vi "find.vi"() -> ()   [LabVIEW 2013]
uses:
  newCore/Variables/GlobalConAxisPI.vi
  newCore/Camera/lib/System Files/user.lib/atmcd32d.llb/Shutter_type typedef.ctl
  newCore/Camera/lib/System Files/user.lib/atmcd32d.llb/Shutter_mode typedef.ctl
  newCore/Camera/vi/GlobalSetGetConfigureCamera.vi
  newCore/Camera/vi/ccdChipPixels.vi
  <vilib>/vision/Image Controls.llb/IMAQ Rounding Mode.ctl
  newCore/Variables/patternImg.vi
  <vilib>/vision/Pattern Matching.llb/IMAQ Match Range Setting.ctl
  <vilib>/vision/Pattern Matching.llb/IMAQ Curve Parameters.ctl
panel:
  in  "Tab Control":T1(tab)
  out "Histogram":i32[][](graph)
  out "Trace":i32[][](graph)=[[2, 0, 0, 1, 1, 1, 0, 0, 0, 1, 0, 1, 0, 1, 2, 2, 0, 3, 0, 2, 2, 1, 3, 1, 0, 1, 1, 1, 0, 1, 3, 1, 0, 2, 0, 1, 0, 1, 1, 0, 1, 1, 3, 1, 0, 2, 0, 1, 1, 0, 0, 2, 0, 0, 1, 1, 1, 0, 0, 1, 0, 1, 0, 0, 0, 1, 2, 1, 1, 2, 0, 2, 4, 3, 1, 1, 0, 0, 1, 1, 2, 0, 1, 1, 0, 0, 0, 1, 1, 1, 1, 3, 0, 0, 1, 0, 0, 0, 2, 1, 1, 1, 2, 1, 0, 1, 1, 0, 0, 2, 1, 1, 0, 0, 1, 1, 1, 1, 0, 2, 2, 0, 1, 2, 1, 0, 3, 0, 2, 1, 3, 0, 1, 1, 0, 0, 3, 0, 0, 0, 0, 0, 0, 0, 0, 0, 0, 0, 0, 0, 0, 0, 0, 0, 0, 0, 0, 0, 0, 0, 0, 0, 0, 0, 0, 0, 0, 0, 0, 0, 0, 0, 0, 0, 0, 0, 0, 0, 0, 0, 0, 0, 0, 0, 0, 0, 0, 0, 0, 0, 0, 0, 0, 0, 0, 0, 0, 0, 0, 0], [1, 2, 2, 0, 0, 0, 1, 2, 1, 2, 1, 1, 1, 0, 0, 0, 3, 1, 0, 1, 0, 2, 0, 2, 1, 1, 0, 0, 1, 0, 1, 2, 1, 0, 0, 0, 0, 0, 1, 0, 1, 0, 2, 0, 1, 0, 0, 0, 0, 1, 1, 3, 0, 0, 0, 2, 0, 0, 2, 0, 1, 1, 0, 0, 2, 0, 2, 1, 0, 1, 1, 0, 1, 1, 0, 0, 0, 1, 0, 0, 1, 0, 0, 0, 0, 1, 0, 1, 1, 1, 1, 0, 0, 0, 1, 1, 1, 0, 1, 0, 0, 0, 1, 1, 1, 0, 0, 1, 1, 3, 1, 0, 0, 0, 0, 0, 0, 0, 1, 2, 1, 0, 0, 0, 2, 3, 3, 2, 0, 1, 1, 1, 0, 0, 4, 0, 1, 2, 0, 0, 0, 2, 0, 0, 0, 0, 0, 0, 0, 0, 0, 0, 0, 0, 0, 0, 0, 0, 0, 0, 0, 0, 0, 0, 0, 0, 0, 0, 0, 0, 0, 0, 0, 0, 0, 0, 0, 0, 0, 0, 0, 0, 0, 0, 0, 0, 0, 0, 0, 0, 0, 0, 0, 0, 0, 0, 0, 0, 0, 0], [2, 2, 0, 1, 2, 0, 1, 0, 2, 3, 1, 0, 1, 0, 1, 0, 0, 0, 0, 2, 1, 0, 0, 2, 2, 0, 0, 0, 3, 0, 0, 2, 2, 2, 0, 3, 0, 3, 1, 3, 1, 3, 1, 0, 3, 1, 3, 3, 1, 1, 1, 1, 2, 0, 1, 0, 1, 1, 1, 3, 0, 2, 3, 1, 1, 1, 0, 1, 0, 1, 2, 3, 1, 2, 1, 3, 0, 2, 0, 2, 0, 1, 0, 2, 2, 1, 1, 3, 1, 2, 1, 1, 1, 3, 0, 0, 0, 0, 1, 1, 1, 0, 1, 0, 2, 1, 1, 0, 1, 0, 1, 2, 2, 2, 2, 0, 1, 0, 0, 0, 1, 1, 2, 0, 0, 1, 5, 2, 2, 0, 2, 0, 2, 2, 2, 0, 1, 0, 6, 0, 0, 0, 0, 0, 0, 0, 0, 0, 0, 0, 0, 0, 0, 0, 0, 0, 0, 0, 0, 0, 0, 0, 0, 0, 0, 0, 0, 0, 0, 0, 0, 0, 0, 0, 0, 0, 0, 0, 0, 0, 0, 0, 0, 0, 0, 0, 0, 0, 0, 0, 0, 0, 0, 0, 0, 0, 0, 0, 0, 0], [0, 0, 1, 0, 1, 1, 0, 0, 0, 1, 1, 0, 1, 0, 0, 0, 0, 0, 2, 0, 0, 0, 0, 2, 0, 0, 0, 1, 1, 2, 1, 1, 1, 2, 1, 0, 0, 3, 0, 1, 1, 0, 0, 0, 0, 1, 0, 0, 2, 1, 0, 0, 1, 1, 1, 2, 2, 0, 1, 0, 0, 1, 0, 1, 1, 0, 0, 2, 1, 1, 2, 1, 1, 0, 0, 0, 0, 2, 1, 0, 0, 0, 0, 1, 0, 1, 0, 0, 0, 0, 1, 0, 0, 0, 0, 1, 0, 1, 1, 1, 0, 2, 3, 1, 1, 0, 1, 1, 1, 0, 1, 0, 0, 1, 1, 0, 2, 0, 0, 0, 0, 3, 0, 0, 0, 0, 0, 0, 0, 0, 1, 0, 2, 0, 0, 0, 1, 2, 2, 0, 1, 0, 0, 0, 0, 0, 0, 0, 0, 0, 0, 0, 0, 0, 0, 0, 0, 0, 0, 0, 0, 0, 0, 0, 0, 0, 0, 0, 0, 0, 0, 0, 0, 0, 0, 0, 0, 0, 0, 0, 0, 0, 0, 0, 0, 0, 0, 0, 0, 0, 0, 0, 0, 0, 0, 0, 0, 0, 0, 0]]
  out "Point":dbl[][](graph)
  out "Image Out":T2(plugin-control)
  out "Image Number":u32
  out "acquired FPS":dbl
  out "Image":i32[][](graph)
  out "AM image":T2(plugin-control)
  out "Number of Particles":i32
  out "Image 2":dbl[][](graph)
  out "concatenated string":string
  out "Task":T3(ring)
  in  "PI SystemNumber":i32=1
  in  "WS File Tree":string(tree)
  out "Active pt3":path
  out "Workspace":path=path "X:/MTusers/Christoph/2011-02-01 Andi/2011-02-01.msw"
  out "Stop Measurement":bool
  out "Buffer Overrun":bool
  out "Running":bool
  out "Global Stop":bool=TRUE
  out "x-position":dbl format="%.3f"
  out "y-position":dbl format="%.3f"
  out "z-position":dbl format="%.3f"
  out "Auto Meas Progress":i32(slide) caption="Point 34 / 34" scale=0.0..34.0
  out "NxtAutMesPoint":i32
  out "Auto Measure Points":i32
  out "subarray":dbl[](array[numeric])
  out "Pattern":dbl[][](array[numeric])
  in  "Remove Outliers":i32=10
  in  "Filter":bool=TRUE
  in  "Exclude / Include X":bool
  in  "X Start 2":dbl
  in  "X End 2":dbl
  in  "Y Start 2":dbl
  in  "Y End 2":dbl
  in  "Exclude / Include Y":bool
  in  "Measurement Parameter 1":T4 items=["Center of Mass X", "Center of Mass Y", "First Pixel X", "First Pixel Y", "Bounding Rect Left", "Bounding Rect Top", "Bounding Rect Right", "Bounding Rect Bottom", "Max Feret Diameter Start X", "Max Feret Diameter Start Y", "Max Feret Diameter End X", "Max Feret Diameter End Y", "Max Horiz. Segment Length Left", "Max Horiz. Segment Length Right", "Max Horiz. Segment Length Row", "-", "Bounding Rect Width", "Bounding Rect Height", "Bounding Rect Diagonal", "Perimeter", "Convex Hull Perimeter", "Holes' Perimeter", "Max Feret Diameter", "Equivalent Ellipse Major Axis", "Equivalent Ellipse Minor Axis", "Equivalent Ellipse Minor Axis (Feret)", "Equivalent Rect Long Side", "Equivalent Rect Short Side", "Equivalent Rect Diagonal", "Equivalent Rect Short Side (Feret)", "Average Horiz. Segment Length", "Average Vert. Segment Length", "Hydraulic Radius", "Waddel Disk Diameter", "-", "Area", "Holes' Area", "Particle & Holes' Area", "Convex Hull Area", "Image Area", "-", "Number of Holes", "Number of Horiz. Segments", "Number of Vert. Segments", "-", "Orientation", "Max Feret Diameter Orientation", "-", "% Area/Image Area", "% Area/(Particle & Holes' Area)", "Ratio of Equivalent Ellipse Axes", "Ratio of Equivalent Rect Sides", "-", "Elongation Factor", "Compactness Factor", "Heywood Circularity Factor", "Type Factor", "-", "Sum X", "Sum Y", "Sum XX", "Sum XY", "Sum YY", "Sum XXX", "Sum XXY", "Sum XYY", "Sum YYY", "-", "Moment of Inertia XX", "Moment of Inertia XY", "Moment of Inertia YY", "Moment of Inertia XXX", "Moment of Inertia XXY", "Moment of Inertia XYY", "Moment of Inertia YYY", "Norm. Moment of Inertia XX", "Norm. Moment of Inertia XY", "Norm. Moment of Inertia YY", "Norm. Moment of Inertia XXX", "Norm. Moment of Inertia XXY", "Norm. Moment of Inertia XYY", "Norm. Moment of Inertia YYY", "Hu Moment 1", "Hu Moment 2", "Hu Moment 3", "Hu Moment 4", "Hu Moment 5", "Hu Moment 6", "Hu Moment 7"]
  in  "Range Lower Value Par 1":dbl
  in  "Range Upper Value  Par 1":dbl
  in  "Ex/In Par 1":bool
  in  "Measurement Parameter 2":T4 items=["Center of Mass X", "Center of Mass Y", "First Pixel X", "First Pixel Y", "Bounding Rect Left", "Bounding Rect Top", "Bounding Rect Right", "Bounding Rect Bottom", "Max Feret Diameter Start X", "Max Feret Diameter Start Y", "Max Feret Diameter End X", "Max Feret Diameter End Y", "Max Horiz. Segment Length Left", "Max Horiz. Segment Length Right", "Max Horiz. Segment Length Row", "-", "Bounding Rect Width", "Bounding Rect Height", "Bounding Rect Diagonal", "Perimeter", "Convex Hull Perimeter", "Holes' Perimeter", "Max Feret Diameter", "Equivalent Ellipse Major Axis", "Equivalent Ellipse Minor Axis", "Equivalent Ellipse Minor Axis (Feret)", "Equivalent Rect Long Side", "Equivalent Rect Short Side", "Equivalent Rect Diagonal", "Equivalent Rect Short Side (Feret)", "Average Horiz. Segment Length", "Average Vert. Segment Length", "Hydraulic Radius", "Waddel Disk Diameter", "-", "Area", "Holes' Area", "Particle & Holes' Area", "Convex Hull Area", "Image Area", "-", "Number of Holes", "Number of Horiz. Segments", "Number of Vert. Segments", "-", "Orientation", "Max Feret Diameter Orientation", "-", "% Area/Image Area", "% Area/(Particle & Holes' Area)", "Ratio of Equivalent Ellipse Axes", "Ratio of Equivalent Rect Sides", "-", "Elongation Factor", "Compactness Factor", "Heywood Circularity Factor", "Type Factor", "-", "Sum X", "Sum Y", "Sum XX", "Sum XY", "Sum YY", "Sum XXX", "Sum XXY", "Sum XYY", "Sum YYY", "-", "Moment of Inertia XX", "Moment of Inertia XY", "Moment of Inertia YY", "Moment of Inertia XXX", "Moment of Inertia XXY", "Moment of Inertia XYY", "Moment of Inertia YYY", "Norm. Moment of Inertia XX", "Norm. Moment of Inertia XY", "Norm. Moment of Inertia YY", "Norm. Moment of Inertia XXX", "Norm. Moment of Inertia XXY", "Norm. Moment of Inertia XYY", "Norm. Moment of Inertia YYY", "Hu Moment 1", "Hu Moment 2", "Hu Moment 3", "Hu Moment 4", "Hu Moment 5", "Hu Moment 6", "Hu Moment 7"]
  in  "Range Lower Value Par 2":dbl
  in  "Range Upper Value Par 2":dbl
  in  "Ex/In Par 2":bool
  in  "Settings (GeometricMatching)":T7={"Curve Parameters"={"Extraction Mode"=0, "Edge Threshold"=75, "Edge Filter Size"=1, "Min Length"=25, "Row Search Step Size"=15, "Col Search Step Size"=15, "Max Endpoint Gap"=10, "Closed"=FALSE, "Subpixel"=FALSE}, "Match Mode"={"Rotation"=TRUE, "Scale"=FALSE, "Occlusion"=TRUE, "Reserved"=FALSE, "Reserved"=FALSE, "Reserved"=FALSE}, "Range Settings"=[{"Match Constraints"=0, "Min"=0.0, "Max"=360.0}, {"Match Constraints"=2, "Min"=0.0, "Max"=25.0}], "Number of Matches"=5, "Minimum Match Score"=600.0, "SubPixel Accuracy"=FALSE, "Adv. Geometric Match Options 2"=[{"Setup Data Item"=21, "Item Value"=0.0}, {"Setup Data Item"=22, "Item Value"=1.0}]} {"Curve Parameters"."Extraction Mode" items=["Normal", "Uniform Regions"]; "Curve Parameters"."Edge Filter Size" items=["Fine", "Normal", "Contour Tracing"]; "Curve Parameters"."Max Endpoint Gap" min=0; "Curve Parameters"."Col Search Step Size" min=1 max=255 step=1; "Curve Parameters"."Row Search Step Size" min=1 max=255 step=1; "Curve Parameters"."Min Length" min=0; "Curve Parameters"."Edge Threshold" min=1 max=350 step=1; "Range Settings"."Max" format="%.2f"; "Range Settings"."Min" format="%.2f"; "Range Settings"."Match Constraints" items=["Rotation Angle (degrees)", "Scale Factor (%)", "Occlusion (%)"]; "Adv. Geometric Match Options 2"."Setup Data Item" items=["Curve Extraction Mode", "Curve Edge Threshold", "Curve Edge Filter Size", "Min Curve Length", "Curve Row Search Step Size", "Curve Col Search Step Size", "Curve Max Endpoint Gap", "Extract Closed Curves", "Enable Subpixel Curve Extraction", "Enable Correlation Score", "Enable Subpixel Accuracy", "Subpixel Iterations", "Subpixel Tolerance", "Initial Match List Length", "Enable Target Template Curve Score", "Min Match Separation Distance", "Min Match Separation Angle", "Min Match Separation Scale", "Max Match Overlap", "Enable Coarse Result", "Enable Calibration Support", "Enable Contrast Reversal", "Search Strategy", "Refinement Match Factor", "Subpixel Match Factor"]}
  in  "Square/Hexa":bool=TRUE
  in  "Connectivity 4/8":bool
  in  "Manual":bool
  in  "Mode":enum16{"Gauss", "Radial", "Azimuthal"}(ring)
  in  "Focuswidth":dbl
  in  "Detection Modus":u16(ring) items=["Pattern", "Heuristic"]
  in  "NA":dbl
  in  "Measurement Time":i32=60 min=10 format="%.0d s"
  out "Counts":u32[](array[numeric])
  in  "Adjustment":bool
  in  "Autopoint-Autofocus Z":bool=TRUE
  in  "Auto Measurement Time (ms)":i32=60 caption="Measurement Time (s)" min=10
  in  "Auto Defocussed Cam":bool
  in  "Point Defocussed Cam":bool
  in  "X-Position":dbl=48.0021 caption="X" min=0.0 max=200.0 step=0.1 format="%1.3f um"
  in  "Y-Position":dbl=19.9997 caption="Y" min=0.0 max=200.0 step=0.1 format="%1.3f um"
  in  "Z-Position":dbl=69.999 caption="Z" min=0.0 max=200.0 step=0.1 format="%1.3f um"
  in  "Picture size":dbl=10.0 min=0.1 max=200.0 format="%1.1f um"
  in  "Picture size 2":dbl=10.0 min=0.1 max=200.0 format="%1.1f um"
  in  "Pixel time":dbl=3.0 min=0.1 max=100.0 step=0.1 format="%.1f ms"
  in  "Resolution":dbl=0.08 min=0.01 max=10.0 step=0.01 format="%.2f µm"
  in  "Laser  Profile":string="1"
  in  "Save Files":bool=TRUE
  in  "Axis":enum32{"x-y", "x-z", "y-x", "y-z", "z-x", "z-y"}(ring)
  out "Last Image File No":i32=-1
  in  "CFD Settings":T8={"Sync Level"=17, "Sync ZeroX"=0, "Sync Offset"=0, "Chan Settings"=[{"CHx Level"=50, "CHx ZeroX"=10, "CHx Offset"=-22150}, {"CHx Level"=50, "CHx ZeroX"=10, "CHx Offset"=-21850}, {"CHx Level"=75, "CHx ZeroX"=10, "CHx Offset"=-6000}, {"CHx Level"=75, "CHx ZeroX"=10, "CHx Offset"=-5700}]}
  out "Measure. time":dbl format="%7.1f s"
  in  "Laser pulse duration":i32[](array[numeric]) min=2 max=100000 step=1 format="%d µs"
  # "Range"
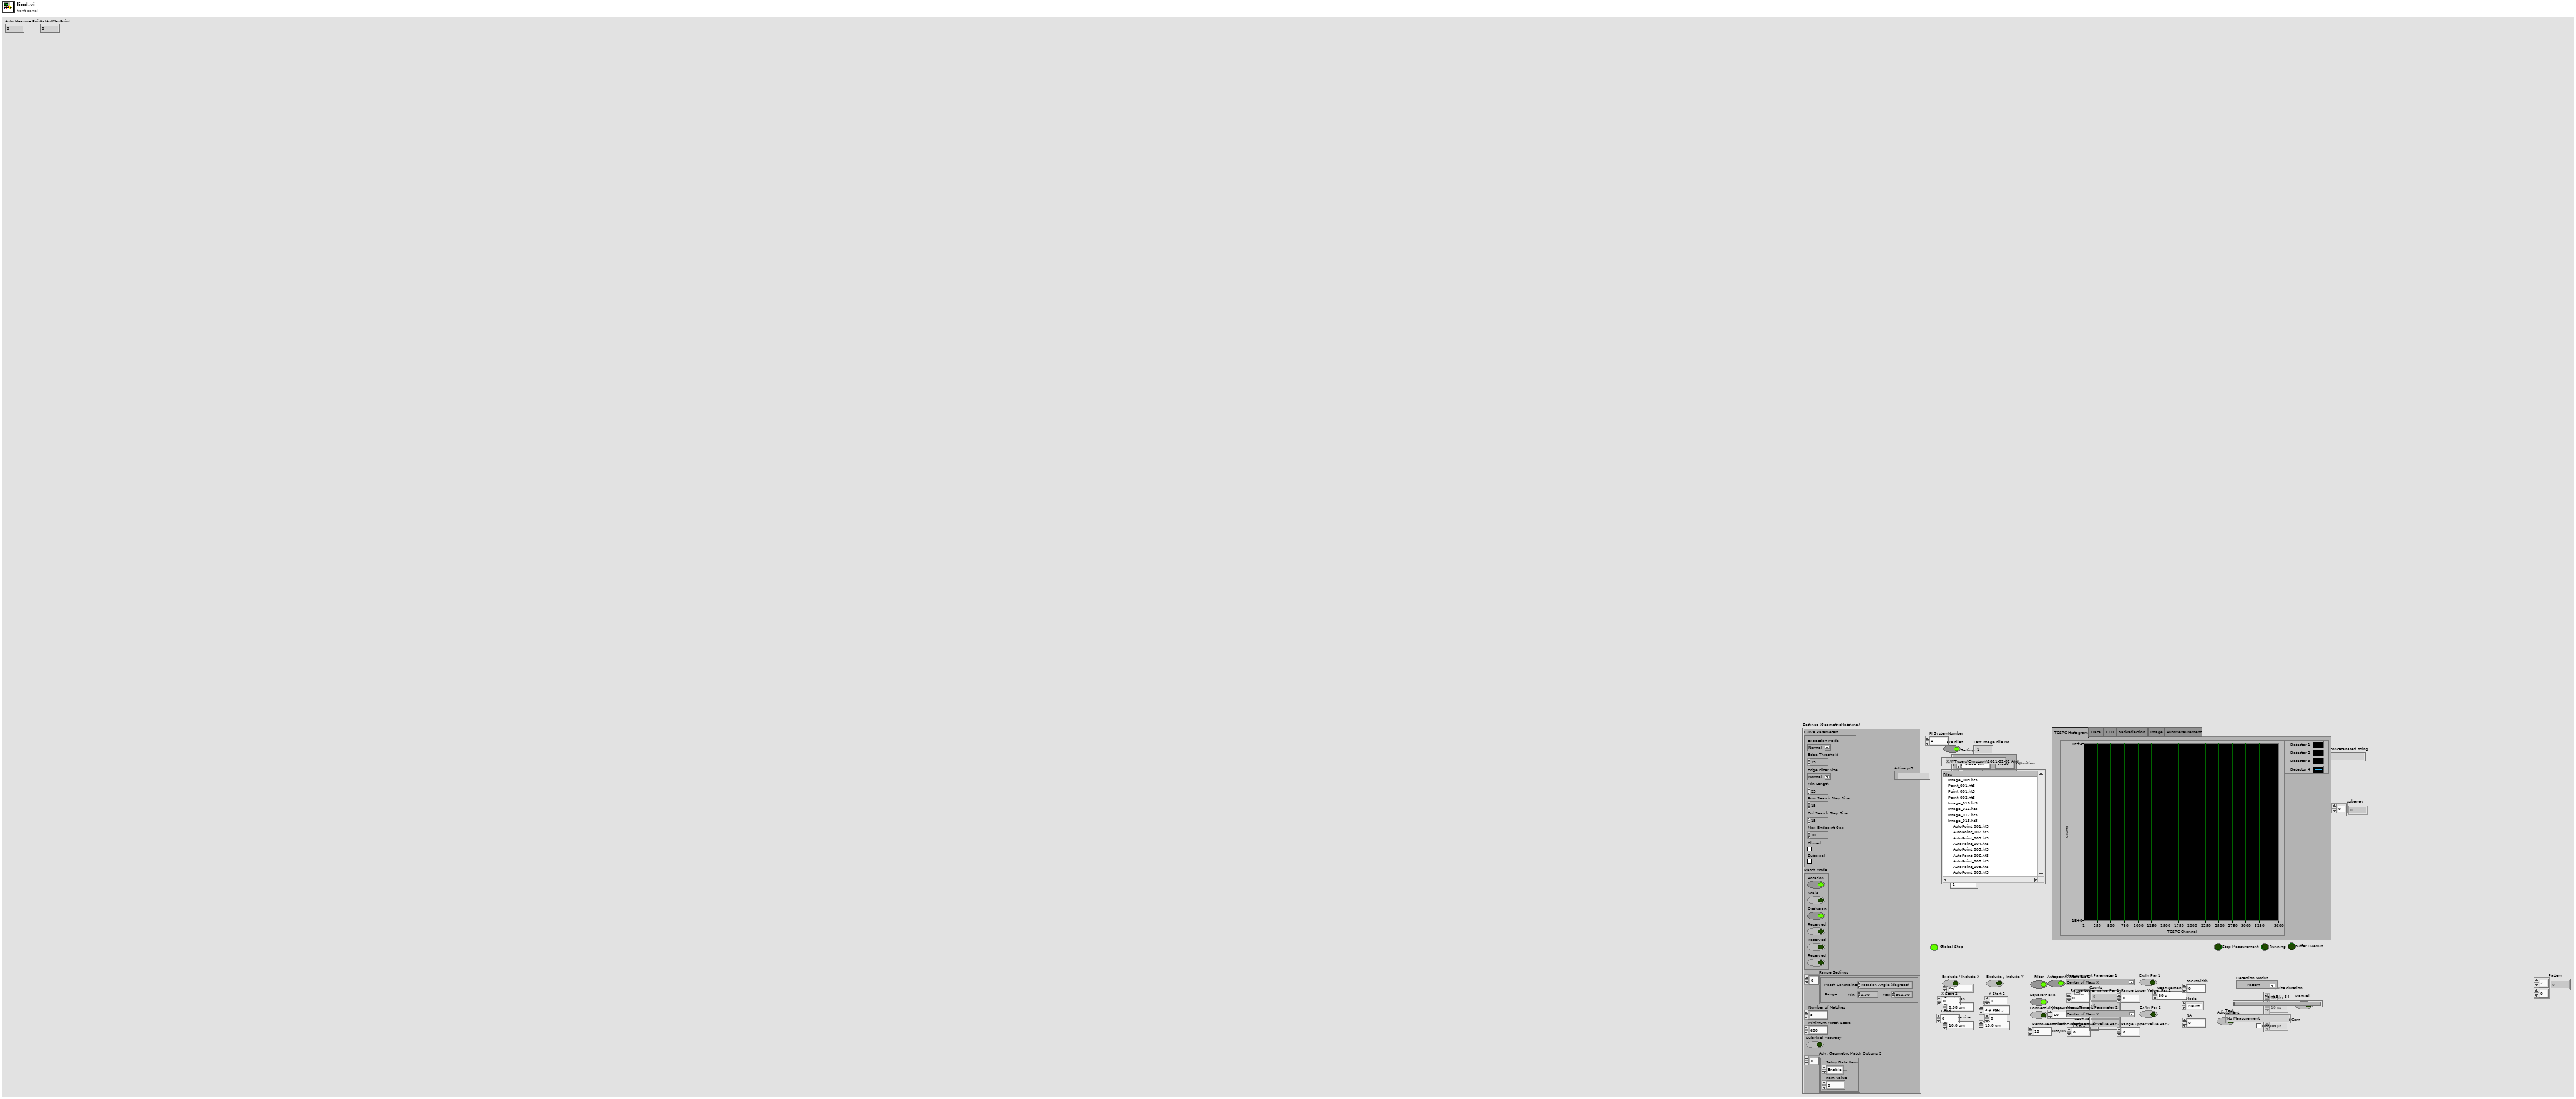
[diagram p1: front panel]
types:
  T1 = enum32{"TCSPC Histogram", "Trace", "CCD", "Backreflection", "Image", "AutoMesaurement"}
  T2 = typedef "IMAQ Image.ctl" = refnum<image>
  T3 = enum16{"No Measurement", "Aquire Image", "Point Measurement", "Multi Measurement", "Save Color Image", "Find Single Mol.", "Auto Measurement Control", "Auto Point", "Aquire Line Scan", "Grid Measurement", "Trapping", "Move Scanner"}
  T4 = typedef "Particle Parameters" = i32
  T5 = typedef "IMAQ Curve Parameters.ctl" = cluster{"Extraction Mode":u32, "Edge Threshold":i32, "Edge Filter Size":u32, "Min Length":i32, "Row Search Step Size":i32, "Col Search Step Size":i32, "Max Endpoint Gap":i32, "Closed":bool, "Subpixel":bool}
  T6 = typedef "IMAQ Match Range Setting.ctl" = cluster{"Match Constraints":u32, "Min":dbl, "Max":dbl}
  T7 = cluster{"Curve Parameters":T5, "Match Mode":cluster{"Rotation":bool, "Scale":bool, "Occlusion":bool, "Reserved":bool, "Reserved":bool, "Reserved":bool}, "Range Settings":T6[], "Number of Matches":i32, "Minimum Match Score":sgl, "SubPixel Accuracy":bool, "Adv. Geometric Match Options 2":cluster{"Setup Data Item":u16, "Item Value":dbl}[]}
  T8 = cluster{"Sync Level":i32, "Sync ZeroX":i32, "Sync Offset":i32, "Chan Settings":cluster{"CHx Level":i32, "CHx ZeroX":i32, "CHx Offset":i32}[]}
  T9 = enum16{"No Measurement", "Aquire Image", "Point Measurement", "Multi Measurement", "Save Color Image", "Find Single Mol.", "Auto Measurement Control", "Auto Point", "Aquire Line Scan", "Grid Measurement"}
  T10 = enum16{"none", "fast axis", "slow axis", "both axis", ""}
  T11 = enum16{"none", "fast axis", "slow axis", "both", ""}
  T12 = enum16{"target position", "relative position", "actual position", "position error"}
  T13 = enum16{"not a pt3 File", "Image File", "Point Measurement", "Auto Point"}
  T14 = enum16{"unknown", "pt3 File", "png Image", "bmp Image"}
  T15 = typedef "Shutter_mode typedef.ctl" = enum16{"Auto", "Open", "Close"}
  T16 = typedef "Shutter_type typedef.ctl" = enum16{"TTL Low", "TTL High"}
  T17 = enum16{"No Measurement", "Aquire Image", "Point Measurement", "Multi Measurement", "Save Color Image", "Find Single Mol.", "Auto Measurement Control", "Auto Point"}
  T18 = typedef "IMAQ Rounding Mode.ctl" = enum16{"Optimize", "Truncate"}
  T19 = cluster{"Measurement Parameter":T4, "Range Lower Value":dbl, "Range Upper Value":dbl, "Range":bool, "Measurement Type":bool}[]
  T20 = enum16{"not a pt3 File", "Image File", "Point Measurement", "Auto Point", "Line Scan"}
  T21 = cluster{"Comment":string, "Binning":i32, "Offset":i32, "AcquisitionTime (ms)":i32, "HardwareSerial":i32, "SyncDivider":i32, "Resolution (ps)":dbl, "CFD Settings":cluster{"Sync Level":i32, "Sync ZeroX":i32, "Sync Offset":i32, "Chan Settings":cluster{"CHx Level":i32, "CHx ZeroX":i32, "CHx Offset":i32}[]}, "ModuleInfo":cluster{"modelcode":i32, "versioncode":i32}[], "BaseResolution (ps)":dbl, "RefClockSource":i32, "ChanInfo":cluster{"CHx Level":i32, "CHx ZeroX":i32, "CHx Offset":i32, "CHx modidx":i32}[], "SyncRate":i32, "InputsEnabled":i64}
  T22 = cluster{"Dimensions":i32, "Time Per Pixel [ms]":dbl, "Acceleration":i32, "Pattern":i32, "X0":sgl, "Y0":sgl, "Z0":dbl, "PixX":i32, "PixY":i32, "PixResol":sgl, "TStartTo":sgl, "TStoptTo":sgl, "TStartFro":sgl, "TStopFro":sgl}
  T23 = cluster{"InpRateFilePos":i64, "StopAfterFilePos":i64}
  T24 = cluster{"X-Position":dbl, "Y-Position":dbl, "Z-Position":dbl}
  T25 = cluster{"File No":i32, "File Path":path, "Parent File":i32, "File Type":enum16{"unknown", "pt3 File", "png Image", "bmp Image"}, "Measurement Type":enum16{"not a pt3 File", "Image File", "Point Measurement", "Auto Point", "Line Scan", "Grid Scan"}, "Upper Left":cluster{"x-Position":dbl, "y-Position":dbl, "z-Position":dbl}, "Pixels":i32[], "Scan Axis":enum32{"x-y", "x-z", "y-z"}, "Resolution":dbl, "PixelTime":dbl}
  T26 = enum16{"not a pt3 File", "Image File", "Point Measurement", "Auto Point", "Line Scan", "Grid Scan"}
  T27 = cluster{"Ident":string, "Format Version":string, "Creator Name":string, "Creator Version":string, "File Time":string, "Comment":string, "Laser":i32, "Binning":i32, "Offset":i32, "AcquisitionTime (ms)":i32, "HardwareSerial":i32, "SyncDivider":i32, "Resolution (ps)":dbl, "Rates":dbl[], "SyncRate":dbl, "CFD Settings":cluster{"Sync Level":i32, "Sync ZeroX":i32, "Sync Offset":i32, "Chan Settings":cluster{"CHx Level":i32, "CHx ZeroX":i32, "CHx Offset":i32}[]}}
  T28 = cluster{"x-Position":dbl, "y-Position":dbl, "z-Position":dbl}
  T29 = typedef "Image Type" = u32
  T30 = cluster{"MesaurementSelection[0]":cluster{"Measurement Parameter":T4, "Range Lower Value":dbl, "Range Upper Value":dbl, "Range":bool, "Measurement Type":bool}, "MesaurementSelection[1]":cluster{"Measurement Parameter":T4, "Range Lower Value":dbl, "Range Upper Value":dbl, "Range":bool, "Measurement Type":bool}, "MesaurementSelection[2]":cluster{"Measurement Parameter":T4, "Range Lower Value":dbl, "Range Upper Value":dbl, "Range":bool, "Measurement Type":bool}, "MesaurementSelection[3]":cluster{"Measurement Parameter":T4, "Range Lower Value":dbl, "Range Upper Value":dbl, "Range":bool, "Measurement Type":bool}, "MesaurementSelection[4]":cluster{"Measurement Parameter":T4, "Range Lower Value":dbl, "Range Upper Value":dbl, "Range":bool, "Measurement Type":bool}, "MesaurementSelection[5]":cluster{"Measurement Parameter":T4, "Range Lower Value":dbl, "Range Upper Value":dbl, "Range":bool, "Measurement Type":bool}, "MesaurementSelection[6]":cluster{"Measurement Parameter":T4, "Range Lower Value":dbl, "Range Upper Value":dbl, "Range":bool, "Measurement Type":bool}, "MesaurementSelection[7]":cluster{"Measurement Parameter":T4, "Range Lower Value":dbl, "Range Upper Value":dbl, "Range":bool, "Measurement Type":bool}, "MesaurementSelection[8]":cluster{"Measurement Parameter":T4, "Range Lower Value":dbl, "Range Upper Value":dbl, "Range":bool, "Measurement Type":bool}}
  T31 = cluster{"Measurement Parameter":T4, "Range Lower Value":dbl, "Range Upper Value":dbl, "Range":bool, "Measurement Type":bool}
  T32 = typedef "IMAQ Point" = cluster{"X":sgl, "Y":sgl}
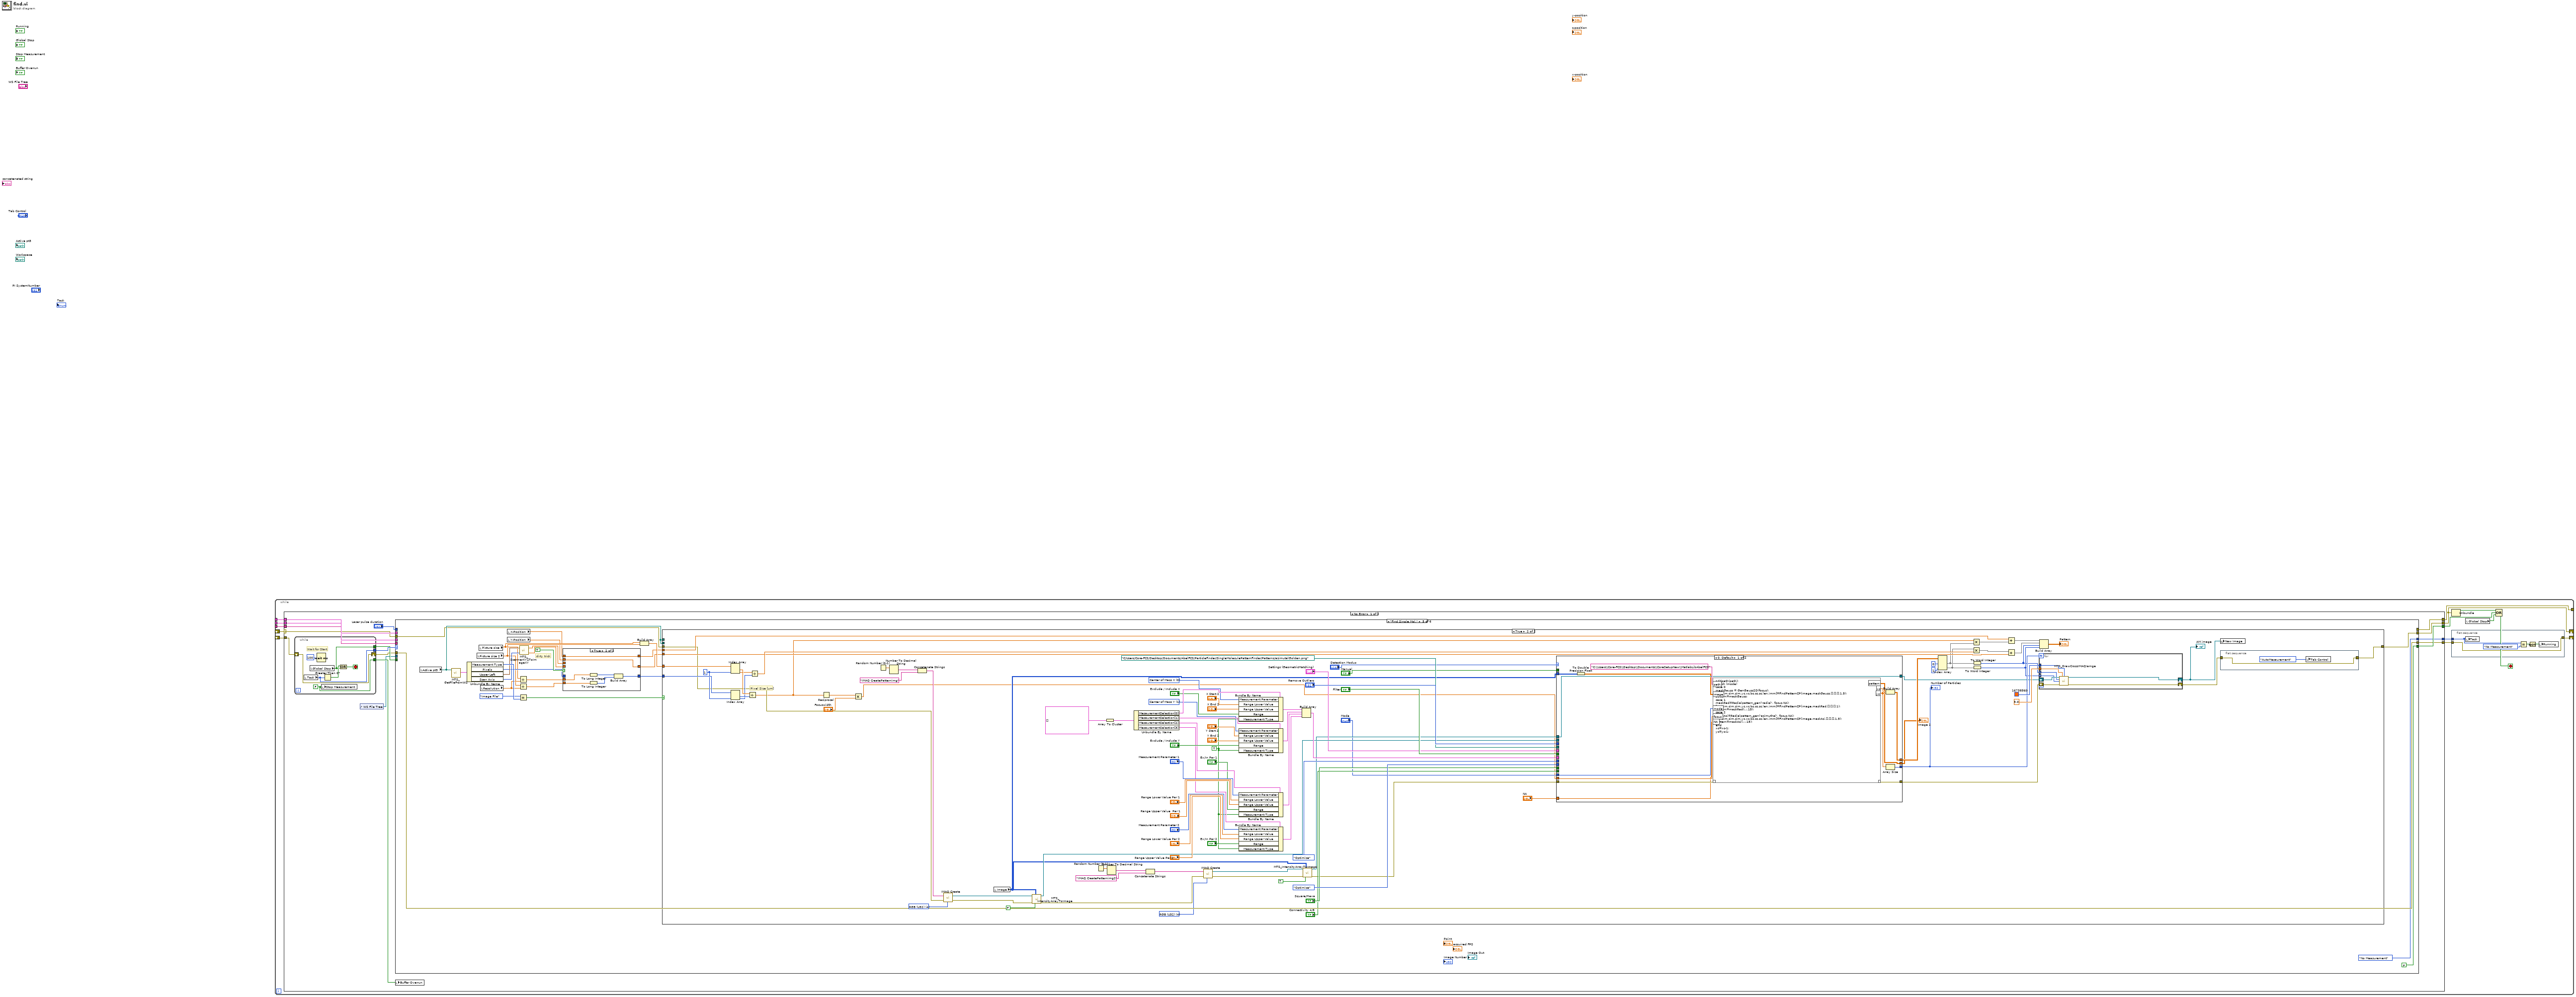
[diagram p0: block diagram]
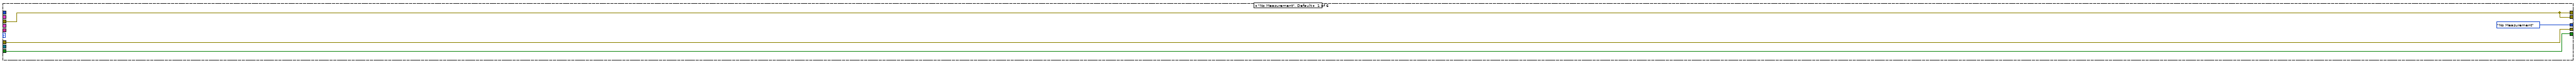
[diagram p2: hidden frame]
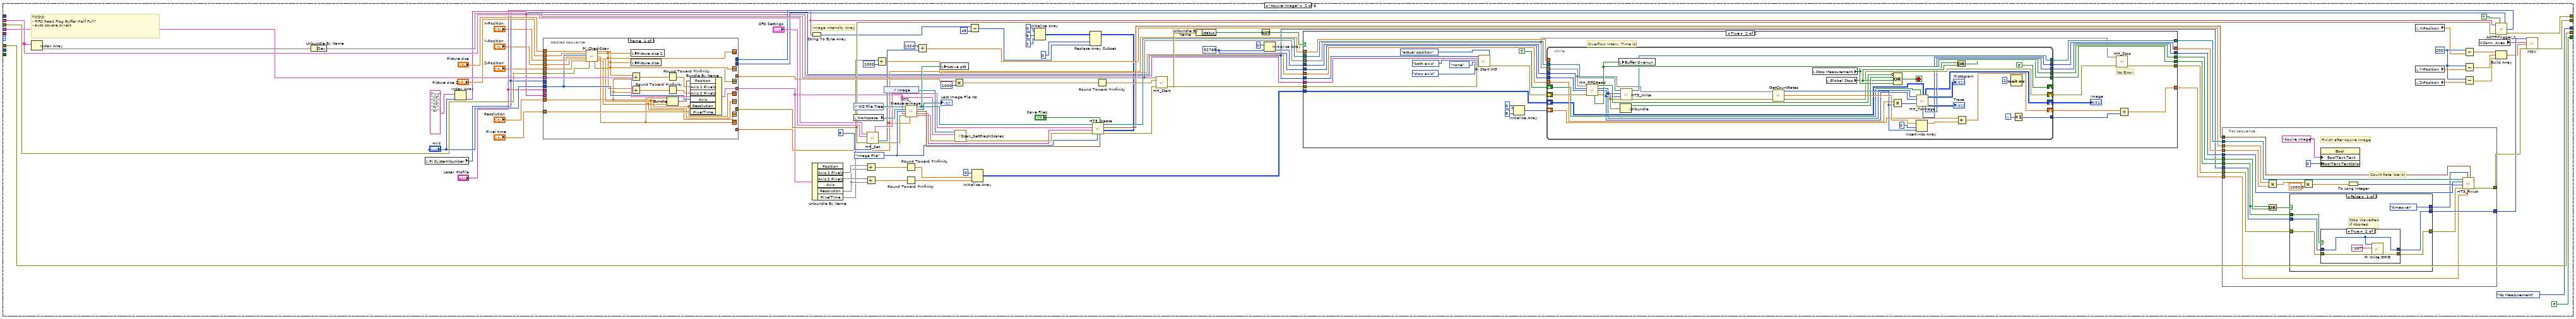
[diagram p3: hidden frame]
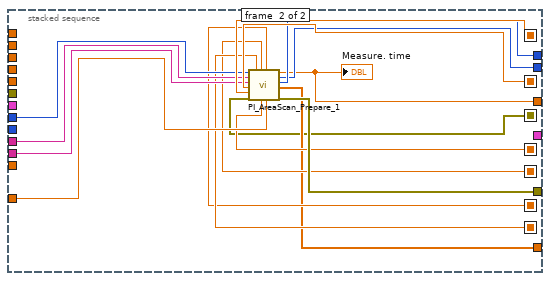
[diagram p4: hidden frame]
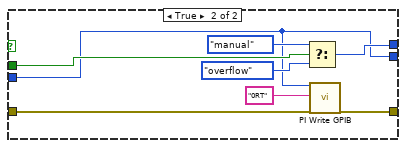
[diagram p6: hidden frame]
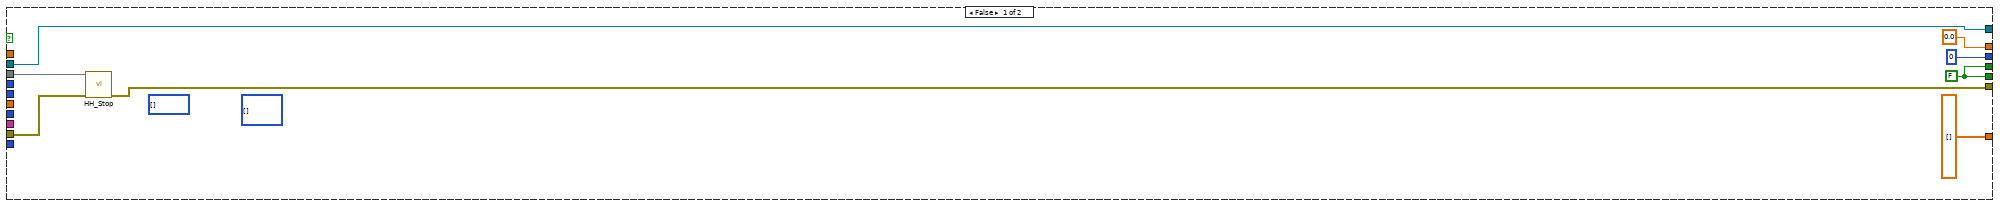
[diagram p7: hidden frame]
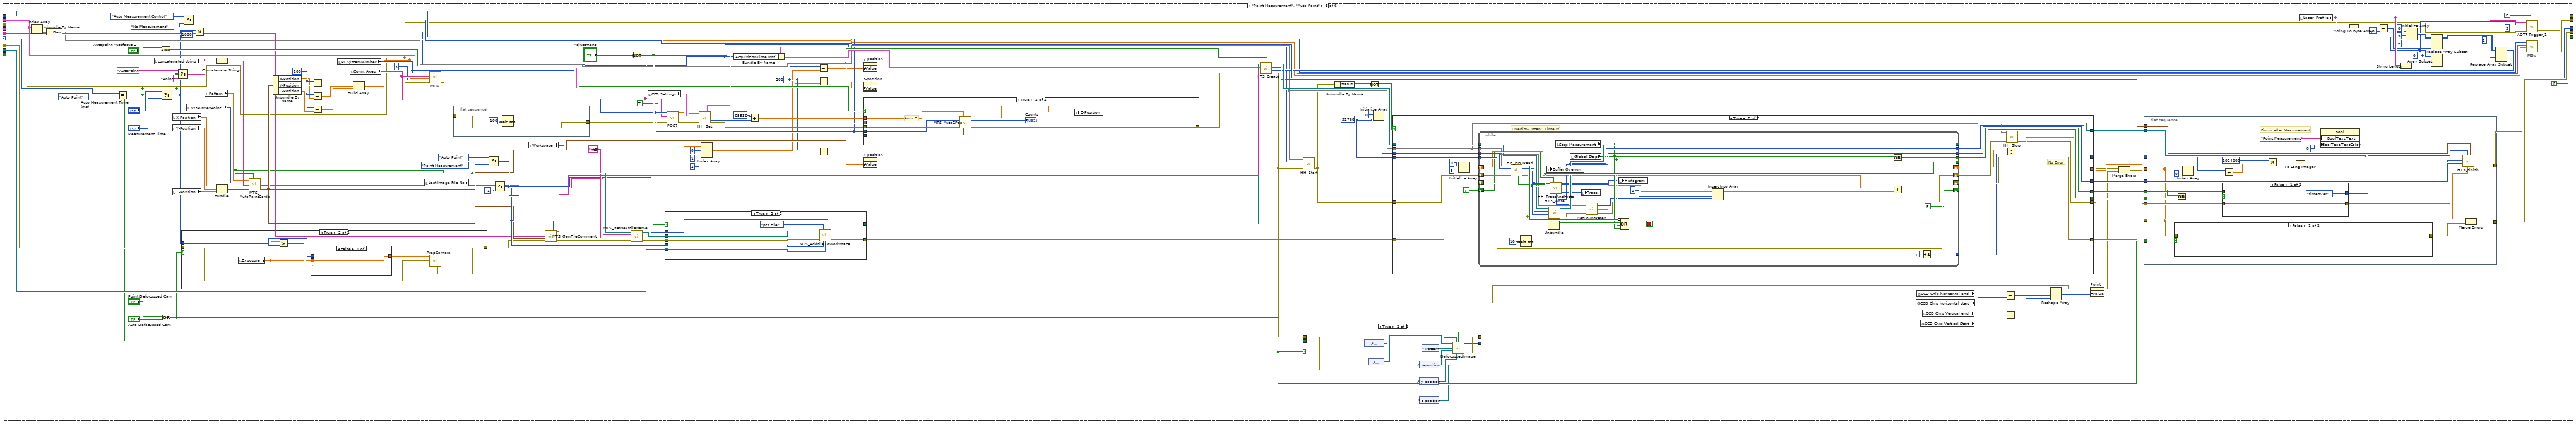
[diagram p8: hidden frame]
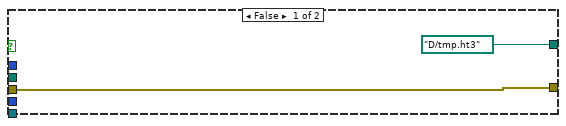
[diagram p12: hidden frame]
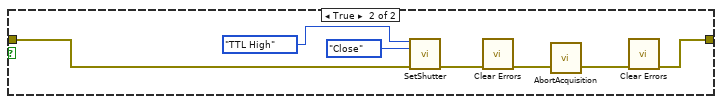
[diagram p14: hidden frame]
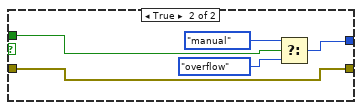
[diagram p15: hidden frame]
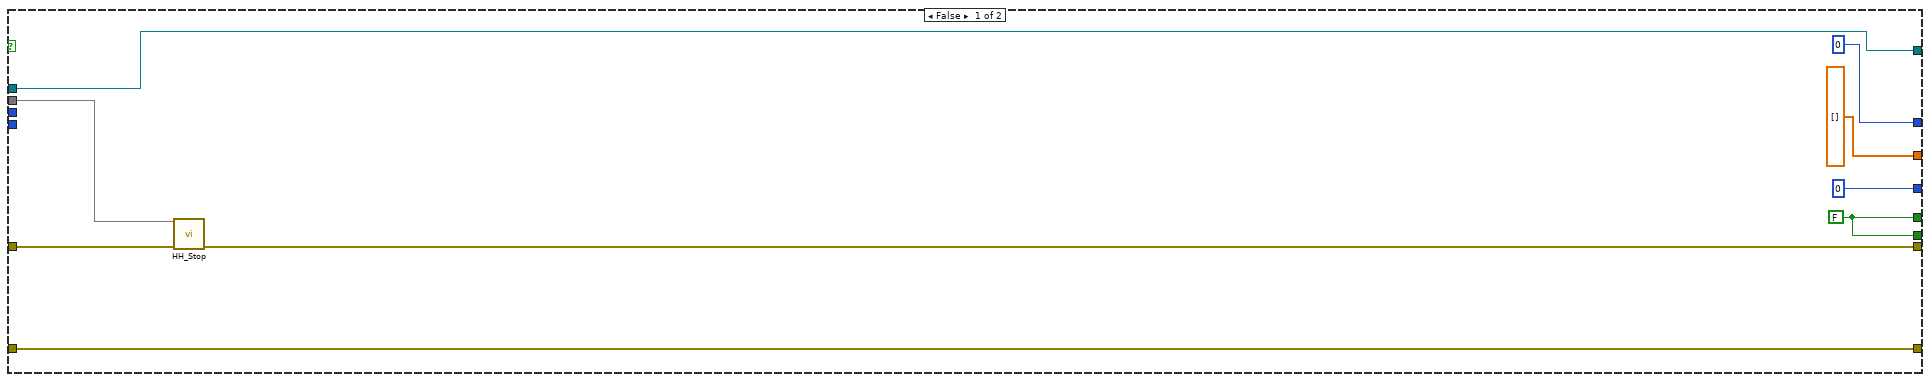
[diagram p16: hidden frame]
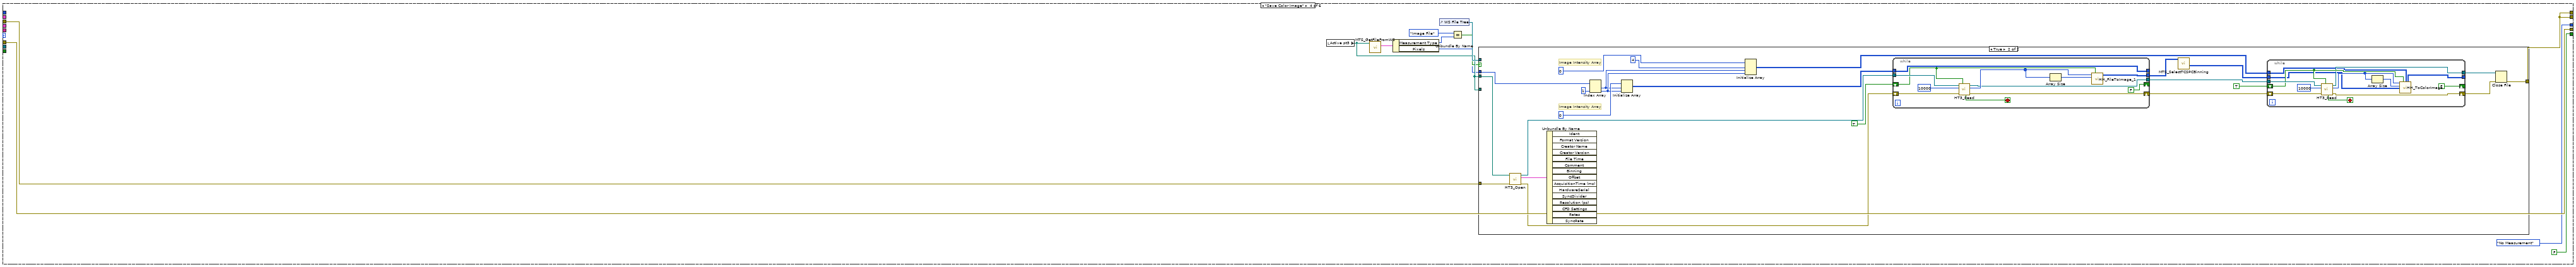
[diagram p17: hidden frame]
diagram:
  n1 = while {
    shift-right: [w7] -> _
    shift-left: _ -> [w4]
    shift-right: [w9] -> _
    shift-left: _ -> [w14]
    tunnel: _ -> [w8]
    tunnel: _ -> [w3]
    tunnel: [w2] -> _
    tunnel: _ -> [w1]
    stop <- w12 stop-if-true
    n2 = case shown="No Error" w4 {
      selector: w4 -> [w20 w890]
      tunnel: w14 -> [w30 w892]
      tunnel: [w29 TRUE ("Global Stop")] -> w11
      tunnel: [w25 w892] -> w10
      tunnel: w8 -> [w24 _]
      tunnel: [w23 w890] -> w7
      tunnel: [w21 T9."No Measurement" ("Do Measurement")] -> w5
      tunnel: w3 -> [w18 _]
      tunnel: [w17 w890] -> w2
      tunnel: w1 -> [w15 _]
      frame No Error {
        n3 = while {
          shift-right: [w888] -> w26
          shift-left: w30 -> [w888]
          tunnel: [w883] -> w28
          tunnel: [w885] -> w27
          tunnel: [w884] -> w22
          stop <- w889 stop-if-true
          w884 = FALSE ("FiFo Overrun")
          # "Wait for Start"
          n4 = local read "Task"() -> (w883:T3)
          n5 = local read "Global Stop"() -> (w885:bool)
          n6 = Wait (ms)(milliseconds to wait=u32 100) -> ()  [unwired: 1 out]
          n7 = local write "Stop Measurement"(w884) -> ()
          n8 = Greater Than 0?(x=w883) -> (x > 0?=w887:bool)
          n9 = Or(x=w887, y=w885) -> (x .or. y?=w889:bool)
        }
        n10 = control-ref of="WS File Tree"() -> (w19:refnum<vi>)
        n11 = case shown="\"Find Single Mol.\"" w28 {
          selector: w28 -> [_ _ w396 _ _ _]
          tunnel: w20 -> [w31 w79 w304 w578 w647 w846]
          tunnel: [w31 w49 w352 w567 w645 w846] -> w23
          tunnel: [w32 FALSE ("Global Stop") FALSE ("Global Stop") FALSE ("Global Stop") FALSE ("Global Stop") FALSE ("Global Stop")] -> w29
          tunnel: w27 -> [w32 _ _ _ _ _]
          tunnel: w26 -> [w34 w63 w303 w577 w646 w847]
          tunnel: [w34 w63 w417 w577 w646 w845] -> w25
          tunnel: w24 -> [_ w129 w354 _ _ _]
          tunnel: [T9."No Measurement" ("Do Measurement") T9."No Measurement" ("Do Measurement") w395 T9."No Measurement" ("Do Measurement") T17."No Measurement" ("Do Measurement") w844] -> w21
          tunnel: w19 -> [_ _ w385 _ _ _]
          tunnel: w18 -> [_ w107 _ _ _ _]
          tunnel: [w31 w81 w378 w567 _ _] -> w17
          tunnel: "Laser pulse duration" -> [_ _ w360 _ _ _]
          tunnel: w15 -> [_ _ w351 _ _ _]
          frame "No Measurement", Default {
          }
          frame "Aquire Image" {
            w42 = 200
            w73 = T20."Image File" ("Measurement Type")
            w110 = 32768 ("dimension size")
            # "TODO:\n- FIFO Read Flag Buffer Half Full?\n- auto square pixels"
            # "Image Intensity Array"
            n12 = Index Array(array=w129) -> (element=w128)  [unwired: 1 in]
            n13 = Unbundle By Name(w128) -> ("Dev"=w101)
            n14 = local read "PI SystemNumber"() -> (w51:i32)
            n15 = Index Array(array=string[] ["yx", "yz", "xy", "xz", "zy", "zx"] ("Array"), index="Axis") -> (element=w56:string)
            n16 = stacked-sequence {
              seq-local: [w141 _] -> [_ w168]
              seq-local: [w140 _] -> [_ w169]
              seq-local: [w139 _] -> [_ w164]
              seq-local: [w135 _] -> [_ w162]
              seq-local: [w134 _] -> [_ w161]
              seq-local: [w133 _] -> [_ w160]
              seq-local: [w136 _] -> [_ w156]
              tunnel: "Picture size" -> [w154 _]
              tunnel: "Picture size 2" -> [w153 _]
              tunnel: w107 -> [w152 _]
              tunnel: "X-Position" -> [w151 _]
              tunnel: "Y-Position" -> [w150 _]
              tunnel: "Z-Position" -> [w149 _]
              tunnel: "Axis" -> [w143 _]
              tunnel: "Resolution" -> [w139 _]
              tunnel: [w142 _] -> w35
              tunnel: [_ w170] -> w80
              tunnel: w79 -> [w137 _]
              tunnel: w56 -> [_ w167]
              tunnel: "Laser  Profile" -> [_ w166]
              tunnel: "Pixel time" -> [w138 w165]
              tunnel: w51 -> [_ w163]
              tunnel: [_ w155] -> w76
              tunnel: [_ w159] -> w75
              tunnel: [_ w158] -> w74
              tunnel: [_ w157] -> w66
              frame #0 {
                n17 = call "PI_CheckScan.vi"("Picture size"=w154, "Picture size 2"=w153, "Axis"=w143, "x-Position"=w151, "y-Position"=w150, "z-Position"=w149, "error in (no error)"=w137) -> ("error out"=w136:errorcluster, "Picture size out"=w140:dbl, "Picture size out 2"=w141:dbl, "a0"=w135:dbl, "b0"=w134:dbl, "c0"=w133:dbl)  [unwired: 7 in]
                n18 = Divide(x=w140, y=w139) -> (x/y=w146:dbl)
                n19 = Divide(x=w141, y=w139) -> (x/y=w147:dbl)
                n20 = local write "Picture size 2"(w141) -> ()
                n21 = local write "Picture size"(w140) -> ()
                n22 = Round Toward +Infinity(x=w146) -> (ceil(x): smallest int >= x=w145:dbl)
                n23 = Round Toward +Infinity(x=w147) -> (ceil(x): smallest int >= x=w144:dbl)
                n24 = Bundle("a0"=w135, "b0"=w134, "c0"=w133) -> (w148:cluster{"a0":dbl, "b0":dbl, "c0":dbl})  [unwired: 1 in]
                n25 = Bundle By Name(cluster=w152, "Position"=w148, "Axis 1 Pixels"=w145, "Axis 2 Pixels"=w144, "Axis"=w143, "Resolution"=w139, "PixelTime"=w138) -> (w142:cluster{})
              }
              frame #1 {
                n26 = call "PI_AreaScan_Prepare_1.vi"("System"=w163, "Laser"=w166, "Axis"=w167, "da"=w169, "db"=w168, "error in (no error)"=w156, "a0"=w162, "b0"=w161, "Resolution"=w164, "c0"=w160, "Pixel time"=w165) -> ("Tacq"=w155:dbl, "lp"=w158:i32, "ap"=w159:i32, "Trigger"=w157:dbl[], "error out"=w170:errorcluster)  [unwired: 4 in]
                "Measure. time" <- w155
              }
            }
            n27 = String To Byte Array(string="Laser  Profile") -> (unsigned byte array=w58:u8[])
            n28 = Unbundle By Name(w35) -> ("Axis 1 Pixels"=w88, "Axis 2 Pixels"=w89, "Resolution"=w86, "PixelTime"=w70)  [unwired: 2 out]
            n29 = control-ref of="WS File Tree"() -> (w113:refnum<vi>)
            n30 = local read "Workspace"() -> (w118:path)
            n31 = Divide(x=w88, y=w86) -> (x/y=w97:dbl)
            n32 = Divide(x=w89, y=w86) -> (x/y=w99:dbl)
            n33 = call "HH_Set.vi"("Device List"=w129, "CFD Settings"="CFD Settings", "error in (no error)"=w80, "SyncDiv"=8) -> ("ht3 header out"=w93:T21, "Sync Rate"=w91:i32, "error out"=w65:errorcluster)  [unwired: 7 in, 2 out]
            n34 = Divide(x=w70, y=1000) -> (x/y=w68:dbl)
            n35 = control-ref of="Image"() -> (w95:refnum<vi>)
            n36 = Round Toward +Infinity(x=w97) -> (ceil(x): smallest int >= x=w96:dbl)
            n37 = Round Toward +Infinity(x=w99) -> (ceil(x): smallest int >= x=w98:dbl)
            n38 = call "MTS_PreapareImage.vi"("WS File Tree"=w113, "Workspace"=w118, "Measurement Type"=w73, "Image Measurent Parameters"=w35, "error in"=w65, "Trigger"=w66) -> ("File Name (dup)"=w103:path, "File No"=→"Last Image File No":i32, "Image Header"=w105:T22, "Comment"=w106:string, "error out"=w64:errorcluster)  [unwired: 5 in]
            n39 = Divide(x=1024, y=w91) -> (x/y=w72:dbl)
            n40 = local write "Active pt3"(w103) -> ()
            n41 = Multiply(x=w76, y=1000) -> (x*y=w85:dbl)
            n42 = call "Scan_SetGraphScales.vi"("error in (no error)"=w64, "Image Measurent Parameters"=w35, "Image"=w95) -> ("error out"=w94:errorcluster)  [unwired: 8 in]
            n43 = Subtract(x=w58, y=48) -> (x-y=w57:i32[])
            n44 = Initialize Array(0 ("element"), w96, w98) -> (w69:i32[][])
            n45 = Initialize Array(0, 5, 2) -> (w55:i32[][])
            n46 = Replace Array Subset(array=w55, new element=w57, index (col)=0) -> (w53:i32[][])  [unwired: 1 in]
            n47 = call "HT3_Create.vi"("Laser"=w53, "Image Header in"=w105, "Save pt3"="Save Files", "Measurement Type"=w73, "error in"=w94, "Comment"=w106, "ht3 Header in"=w93, "File Path"=w103) -> ("error out"=w119:errorcluster, "FileHeaderPos"=w109:T23, "refnum out"=w117:refnum<file>)  [unwired: 1 in]
            n48 = Round Toward +Infinity(x=w85) -> (ceil(x): smallest int >= x=w83:dbl)
            n49 = call "HH_Start.vi"("Device Index"=w101, "Acq. Time"=w83, "error in (no error)"=w119) -> ("error out"=w126:errorcluster)  [unwired: 11 in, 1 out]
            n50 = Unbundle By Name(w126) -> ("status"=w127:bool)
            n51 = Not(x=w127) -> (.not. x?=w125:bool)
            n52 = Initialize Array(u32 0, w110) -> (w122:u32[])
            n53 = case shown="True" w125 {
              tunnel: [w218 w249] -> w124
              tunnel: w51 -> [_ w244]
              tunnel: w126 -> [w219 w245]
              tunnel: w101 -> [w217 w236]
              tunnel: w69 -> [_ w221]
              tunnel: w122 -> [_ w243]
              tunnel: w110 -> [_ w242]
              tunnel: [w216 w241] -> w121
              tunnel: [w216 w240] -> w120
              tunnel: w117 -> [w215 w239]
              tunnel: [w215 w238] -> w116
              tunnel: [0 ("Num Records Total") w237] -> w115
              tunnel: [0.0 w230] -> w114
              tunnel: w56 -> [_ w233]
              tunnel: [dbl[] [] w227] -> w71
              tunnel: w68 -> [_ w223]
              tunnel: w66 -> [_ w222]
              frame False {
                (unwired) i32[][] [] ("Image Array Out")
                (unwired) u64[] [] ("Histograms")
                w216 = FALSE ("Stop Measurement")
                n54 = call "HH_Stop.vi"("Device Index"=w217, "error in (no error)"=w219) -> ("error out"=w218:errorcluster)  [unwired: 12 in, 1 out]
              }
              frame True {
                # "Overflow Interv. Time (s)"
                # "No Error"
                n55 = call "PI Start WG.vi"("System no."=w244, "axis"=w233, "Generator"=T10."both axis", "Init DDL"=T11."none", "increment"=T11."slow axis", "error in"=w245, "saved data"=T12."actual position") -> ("error out"=w246:errorcluster)  [unwired: 12 in]
                n56 = Initialize Array(0, 5) -> (w224:i32[])
                n57 = while {
                  tunnel: w236 -> [w269]
                  tunnel: w243 -> [w285]
                  tunnel: w242 -> [w284]
                  shift-right: [w270] -> w248
                  shift-left: w246 -> [w286]
                  shift-right: [FALSE ("Reset")] -> _
                  shift-left: TRUE ("Reset") -> [w257]
                  tunnel: [w278] -> w241
                  tunnel: [w274] -> w240
                  tunnel: w239 -> [w276]
                  tunnel: [w275] -> w238
                  tunnel: [w253] -> w237
                  tunnel: [w252] -> w230
                  shift-right: [w266] -> w229
                  shift-left: w224 -> [w264]
                  tunnel: [w263] -> w228
                  tunnel: w223 -> [w260]
                  tunnel: w222 -> [_]
                  shift-right: [w251] -> w220
                  shift-left: w221 -> [w259]
                  i -> [w262]
                  stop <- w283 stop-if-true
                  n58 = call "HH_FIFORead.vi"("Device Index"=w269, "Buffer In"=w285, "Count"=w284, "error in (no error)"=w286) -> ("OK"=w279:bool, "Buffer Out"=w256:u32[], "Data Count"=w255:i32, "FiFo Overrun"=w278:bool, "error out"=w277:errorcluster)  [unwired: 7 in]
                  n59 = local write "Buffer Overrun"(w278) -> ()
                  n60 = Unbundle(w277) -> ("status"=w282:bool)  [unwired: 2 out]
                  n61 = call "HT3_Write.vi"("error in"=w277, "Data Count"=w255, "Data in"=w256, "refnum in"=w276) -> ("error out"=w271:errorcluster, "refnum out"=w275:refnum<file>)  [unwired: 6 in]
                  n62 = call "GetCountRates.vi"("error in (no error)"=w271, "DeviceIndex"=w269) -> ("error out"=w270:errorcluster, "CntRates"=w268:dbl[], "SyncRate"=w261:i32)  [unwired: 1 in]
                  n63 = local read "Stop Measurement"() -> (w273:bool)
                  n64 = local read "Global Stop"() -> (w272:bool)
                  n65 = Multiply(x=w260, y=w261) -> (x*y=w250:i32)
                  n66 = Compound Arithmetic op=OR(invert w279, w282, w272, w273) -> (w283:bool)
                  n67 = Insert Into Array(array=w268, index=0, new element=w261) -> (w265:dbl[])
                  n68 = call "HH_ToImage.vi"("Data In"=w256, "Reset"=w257, "Image Array In"=w259, "Data Count"=w255, "Pixel Time (Laser Pulses)"=w250) -> ("Image Array Out"=w251:i32[][], "Histograms"=→"Histogram":i32[][], "Total Oveflow Count"=w252:u64, "Num Records Total"=w253:i64, "Traces"=→"Trace":i32[][])  [unwired: 4 in, 2 out]
                  n69 = Or(x=w273, y=w272) -> (x .or. y?=w274:bool)
                  n70 = Add(x=w264, y=w265) -> (x+y=w266:dbl[])
                  n71 = Wait (ms)(milliseconds to wait=u32 2) -> ()  [unwired: 1 out]
                  n72 = Increment(x=w262) -> (x+1=w263:i32)
                }
                "Image" <- w220
                n73 = call "HH_Stop.vi"("Device Index"=w236, "error in (no error)"=w248) -> ("error out"=w249:errorcluster)  [unwired: 12 in, 1 out]
                n74 = Divide(x=w229, y=w228) -> (x/y=w227:dbl[])
              }
            }
            n75 = flat-sequence {
              tunnel: w124 -> [w189]
              tunnel: [w178] -> w50
              tunnel: w121 -> [w191]
              tunnel: w120 -> [w180]
              tunnel: w51 -> [w188]
              tunnel: [w187] -> w48
              tunnel: w116 -> [w185]
              tunnel: w115 -> [w184]
              tunnel: w114 -> [w174]
              tunnel: w109 -> [w179]
              tunnel: w72 -> [w175]
              tunnel: w71 -> [w171]
              frame #0 {
                # "Count Rate (per s)"
                # "Finish after Aquire Image"
                n76 = Multiply(x=w175, y=w174) -> (x*y=w173:dbl)
                n77 = Or(x=w180, y=w191) -> (x .or. y?=w190:bool)
                n78 = case shown="False" w190 {
                  tunnel: w189 -> [w196 w206]
                  tunnel: w188 -> [w194 w207]
                  tunnel: [w193 w207] -> w187
                  tunnel: [w195 w205] -> w186
                  tunnel: [enum16{"timeover", "manual", "overflow"}."timeover" ("Stop Reason") w210] -> w181
                  tunnel: w180 -> [w192 w208]
                  frame False {
                    # "Stop WaveGen\nif Aborted"
                    n79 = case shown="True" w192 {
                      tunnel: w196 -> [w198 w203]
                      tunnel: [w198 w202] -> w195
                      tunnel: w194 -> [w199 w201]
                      tunnel: [w199 w201] -> w193
                      frame False {
                      }
                      frame True {
                        n80 = call "PI Write GPIB.vi"("System no."=w201, "String to send"="0RT", "error in"=w203) -> ("error out"=w202:errorcluster)  [unwired: 16 in]
                      }
                    }
                  }
                  frame True {
                    n81 = Select(t=enum16{"timeover", "manual", "overflow"}."manual" ("Stop Reason"), s=w208, f=enum16{"timeover", "manual", "overflow"}."overflow" ("Stop Reason")) -> (s? t:f=w210:enum16{"timeover", "manual", "overflow"})
                    n82 = call "PI Write GPIB.vi"("System no."=w207, "String to send"="0RT", "error in"=w206) -> ("error out"=w205:errorcluster)  [unwired: 16 in]
                  }
                }
                n83 = Multiply(x=w173, y=1000.0) -> (x*y=w183:dbl)
                n84 = property on="Property Node" class="Bool"("BoolText.Text"="Aquire Image" ("Caption.Text"), "BoolText.TextColor"=u32 0 ("Boolean Text.Colors:FG Color")) -> ()  [unwired: 2 in, 2 out]
                n85 = To Long Integer(number=w183) -> (32bit integer=w182:i32)
                n86 = call "HT3_Finish.vi"("FileHeaderPos"=w179, "Rates"=w171, "Stop Reason"=w181, "error in"=w186, "Num Records"=w184, "Stop After (ms)"=w182, "refnum in"=w185) -> ("error out"=w178:errorcluster)  [unwired: 4 in]
              }
            }
            n87 = local read "X-Position"() -> (w41:dbl)
            n88 = local read "Y-Position"() -> (w40:dbl)
            n89 = local read "Z-Position"() -> (w39:dbl)
            n90 = Subtract(x=w42, y=w41) -> (x-y=w38:dbl)
            n91 = Subtract(x=w42, y=w40) -> (x-y=w37:dbl)
            n92 = Subtract(x=w42, y=w39) -> (x-y=w36:dbl)
            n93 = global read "GlobalConAxisPI.vi" "Conn. Axes"() -> (w47:string[])
            n94 = call "AOTF-Trigger_1.vi"("Channel"="Laser  Profile", "error in (no error)"=w80, "Triggered"=TRUE, "lp"=w74, "ap"=w75) -> ("error out"=w81:errorcluster)  [unwired: 2 in]
            n95 = Build Array(w38, w37, w36) -> (w46:dbl[])
            n96 = call "MOV.vi"("System no."=w48, "Axes to move"=w47, "Position values"=w46, "error in"=w50) -> ("error out"=w49:errorcluster)  [unwired: 15 in]
          }
          frame "Point Measurement", "Auto Point" {
            w322 = 200
            w327 = 200
            w355 = 0
            w383 = 32768 ("dimension size")
            n97 = Index Array(array=w354) -> (element=w421)  [unwired: 1 in]
            n98 = Unbundle By Name(w421) -> ("Dev"=w340)
            n99 = Equal?(x=w396, y=T3."Auto Point" ("Task")) -> (x = y?=w292:bool)
            n100 = local read "concatenated string"() -> (w347:string)
            n101 = And(x=w292, y="Autopoint-Autofocus Z") -> (x .and. y?=w384:bool)
            n102 = Or(x="Point Defocussed Cam", y="Auto Defocussed Cam") -> (x .or. y?=w309:bool)
            n103 = Select(t="Auto Measurement Time (ms)", s=w292, f="Measurement Time") -> (s? t:f=w293:i32)
            n104 = local read "X-Position"() -> (w402:dbl)
            n105 = local read "Y-Position"() -> (w401:dbl)
            n106 = local read "Z-Position"() -> (w337:dbl)
            n107 = Select(t="AutoPoint" ("Measurement Type"), s=w292, f="Point" ("Measurement Type")) -> (s? t:f=w346:string)
            n108 = case shown="True" w309 {
              tunnel: [w423 w428] -> w302
              tunnel: w303 -> [w423 w429]
              tunnel: w293 -> [_ w426]
              frame False {
              }
              frame True {
                n109 = global read "GlobalSetGetConfigureCamera.vi" "Exposure"() -> (w424:sgl)
                n110 = Greater?(x=w424, y=w426) -> (0:w427:bool)
                n111 = case shown="False" w427 {
                  tunnel: w426 -> [_ w431]
                  tunnel: [w430 w431] -> w425
                  tunnel: w424 -> [w430 _]
                  frame False {
                  }
                  frame True {
                  }
                }
                n112 = call "PrepCamera.vi"("mesTime"=w425, "error out 2"=w429) -> ("error out"=w428:errorcluster)  [unwired: 25 in]
              }
            }
            n113 = Select(t=T3."Auto Measurement Control" ("Task"), s=w292, f=T9."No Measurement" ("Do Measurement")) -> (s? t:f=w395:T3)
            n114 = local read "NxtAutMesPoint"() -> (w341:i32)
            n115 = Multiply(x=w293, y=1000) -> (x*y=w294:i32)
            n116 = local read "Pattern"() -> (w342:dbl[][])
            n117 = Concatenate Strings(w347, w346) -> (w345:string)
            n118 = Bundle("X-Position"=w402, "Y-Position"=w401, "Z-Position"=w337) -> (w386:T24)  [unwired: 1 in]
            n119 = call "MTS_AutoPointCords.vi"("Is Auto Point"=w292, "Cords In"=w386, "Next Auto Measure Point"=w341, "Pattern"=w342) -> ("Cords"=w373:T24)  [unwired: 7 in]
            n120 = Unbundle By Name(w373) -> ("X-Position"=w313:dbl, "Y-Position"=w314:dbl, "Z-Position"=w323:dbl)
            n121 = Subtract(x=w327, y=w314) -> (x-y=w326:dbl)
            n122 = Subtract(x=w327, y=w313) -> (x-y=w325:dbl)
            n123 = Subtract(x=w327, y=w323) -> (x-y=w324:dbl)
            n124 = local read "PI SystemNumber"() -> (w335:i32)
            n125 = global read "GlobalConAxisPI.vi" "Conn. Axes"() -> (w329:string[])
            n126 = Build Array(w326, w325, w324) -> (w328:dbl[])
            n127 = local read "Last Image File No"() -> (w389:i32)
            n128 = call "MOV.vi"("System no."=w335, "Axes to move"=w329, "Position values"=w328, "No.of digits"=i16 3, "error in"=w304) -> ("error out"=w317:errorcluster)  [unwired: 14 in]
            n129 = flat-sequence {
              tunnel: w317 -> [w432]
              tunnel: [w432] -> w316
              frame #0 {
                n130 = Wait (ms)(milliseconds to wait=u32 100) -> ()  [unwired: 1 out]
              }
            }
            n131 = Select(t=T13."Auto Point" ("Measurement Type"), s=w292, f=T13."Point Measurement" ("Measurement Type")) -> (s? t:f=w390:T13)
            n132 = Select(t=w389, s=w292, f=-1) -> (s? t:f=w387:i32)
            n133 = local read "Workspace"() -> (w411:path)
            n134 = call "MTS_GenFileComment.vi"("Measurement Type"=w390, "Parent File No"=w387, "Info"=w351, "Upper Left"=w373, "error in"=w302) -> ("Comment"=w412:string, "error out"=w410:errorcluster)  [unwired: 7 in, 2 out]
            n135 = Not(x="Adjustment") -> (.not. x?=w349:bool)
            n136 = call "MTS_GetNextFileName.vi"("error in (no error)"=w410, "File Type"="ht3", "Measurement Type"=w345, "Workspace"=w411) -> ("error out"=w405:errorcluster, "Next File Name"=w404:path)  [unwired: 6 in]
            n137 = local read "CFD Settings"() -> (w380:T8)
            n138 = case shown="True" w349 {
              tunnel: w405 -> [w446 w454]
              tunnel: w404 -> [_ w453]
              tunnel: [w446 w452] -> w305
              tunnel: [path "D:/tmp.ht3" w447] -> w403
              tunnel: w390 -> [_ w449]
              tunnel: w387 -> [_ w451]
              tunnel: w385 -> [_ w448]
              frame False {
              }
              frame True {
                n139 = call "MTS_AddFileToWorkspace.vi"("File Name"=w453, "File Type"=T14."pt3 File", "Measurement Type"=w449, "error in (no error)"=w454, "Parent"=w451, "Tree Refnum"=w448) -> ("File Name (dup)"=w447:path, "error out"=w452:errorcluster)  [unwired: 7 in, 1 out]
              }
            }
            n140 = call "POS?.vi"("System no."=w335, "Axes to query"=w329, "All axes?"=TRUE, "error in"=w316) -> ("Position"=w333:dbl[], "error out"=w336:errorcluster)  [unwired: 14 in]
            n141 = call "HH_Set.vi"("Device List"=w354, "CFD Settings"=w380, "error in (no error)"=w336) -> ("ht3 header out"=w400:T21, "Sync Rate"=w370:i32, "error out"=w398:errorcluster)  [unwired: 8 in, 2 out]
            n142 = Index Array(array=w333, index #1=0 ("index"), index #2=1 ("index"), index #3=2 ("index")) -> (element #1=w321:dbl, element #2=w320:dbl, element #3=w319:dbl)
            n143 = Bundle By Name(cluster=w400, "AcquisitionTime (ms)"=w294) -> (w399:T21)
            n144 = Divide(x=65536 ("n"), y=w370) -> (x/y=w371:dbl)
            n145 = Subtract(x=w322, y=w321) -> (x-y=w291:dbl)
            n146 = Subtract(x=w322, y=w319) -> (x-y=w318:dbl)
            n147 = Subtract(x=w322, y=w320) -> (x-y=w290:dbl)
            n148 = property on="y-position" class="DigNum (strict)"("Value"=w291) -> ()  [unwired: 2 in, 2 out]
            n149 = property on="z-position" class="DigNum (strict)"("Value"=w318) -> ()  [unwired: 2 in, 2 out]
            n150 = case shown="True" w384 {
              tunnel: w398 -> [w455 w463]
              tunnel: [w455 w462] -> w397
              tunnel: w335 -> [_ w457]
              tunnel: w371 -> [_ w461]
              tunnel: w373 -> [_ w460]
              tunnel: w340 -> [_ w456]
              frame False {
              }
              frame True {
                # "Auto Z"
                n151 = call "MTS_AutoZPos.vi"("PH Dev"=w456, "OFlow Interv [s]"=w461, "PI System no."=w457, "error in"=w463, "Start Point"=w460) -> ("New Z"=w459:dbl, "Counts"=→"Counts":u32[], "error out"=w462:errorcluster)  [unwired: 8 in]
                n152 = local write "Z-Position"(w459) -> ()
              }
            }
            n153 = property on="x-position" class="DigNum (strict)"("Value"=w290) -> ()  [unwired: 2 in, 2 out]
            n154 = Initialize Array(u32 0, w383) -> (w415:u32[])
            n155 = global read "ccdChipPixels.vi" "CCD Chip horizontal start"() -> (w300:i32)
            n156 = global read "ccdChipPixels.vi" "CCD Chip horizontal end"() -> (w301:i32)
            n157 = global read "ccdChipPixels.vi" "CCD Chip Vertical Start"() -> (w298:i32)
            n158 = global read "ccdChipPixels.vi" "CCD Chip Vertical end"() -> (w299:i32)
            n159 = Subtract(x=w301, y=w300) -> (x-y=w296:i32)
            n160 = Subtract(x=w299, y=w298) -> (x-y=w295:i32)
            n161 = flat-sequence {
              tunnel: w418 -> [w467]
              tunnel: w306 -> [w484]
              tunnel: [w465] -> w417
              tunnel: [w481] -> w353
              tunnel: w414 -> [w486]
              tunnel: w413 -> [w477]
              tunnel: w407 -> [w480]
              tunnel: w406 -> [w479]
              tunnel: w382 -> [w476]
              tunnel: w375 -> [w473]
              tunnel: w374 -> [w472]
              tunnel: w309 -> [w464]
              frame #0 {
                # "Finish after Measurement"
                n162 = case shown="False" w464 {
                  tunnel: w467 -> [w488 w493]
                  tunnel: [w488 w490] -> w466
                  frame False {
                  }
                  frame True {
                    n163 = call "SetShutter.vi"("type"=Shutter_type_typedef."TTL High", "mode"=Shutter_mode_typedef."Close", "error in (no error)"=w493) -> ("error out"=w495:errorcluster)  [unwired: 11 in, 1 out]
                    n164 = call <vilib>:"Clear Errors.vi"("error in (no error)"=w495) -> ("error out"=w494:errorcluster)  [unwired: 6 in]
                    n165 = call "AbortAcquisition.vi"("error in (no error)"=w494) -> ("error out"=w489:errorcluster)  [unwired: 1 in, 1 out]
                    n166 = call <vilib>:"Clear Errors.vi"("error in (no error)"=w489) -> ("error out"=w490:errorcluster)  [unwired: 6 in]
                  }
                }
                n167 = Or(x=w477, y=w486) -> (x .or. y?=w485:bool)
                n168 = Index Array(array=w473, index=0) -> (element=w474:dbl)
                n169 = case shown="False" w485 {
                  tunnel: w484 -> [w497 w498]
                  tunnel: [w497 w498] -> w482
                  tunnel: [enum16{"timeover", "manual", "overflow"}."timeover" ("Stop Reason") w501] -> w478
                  tunnel: w477 -> [_ w499]
                  frame False {
                  }
                  frame True {
                    n170 = Select(t=enum16{"timeover", "manual", "overflow"}."manual" ("Stop Reason"), s=w499, f=enum16{"timeover", "manual", "overflow"}."overflow" ("Stop Reason")) -> (s? t:f=w501:enum16{"timeover", "manual", "overflow"})
                  }
                }
                n171 = Divide(x=w472, y=w474) -> (x/y=w471:dbl)
                n172 = Multiply(x=1024000, y=w471) -> (x*y=w469:dbl)
                n173 = To Long Integer(number=w469) -> (32bit integer=w468:i32)
                n174 = property on="Property Node" class="Bool"("BoolText.Text"="Point Measurement" ("Caption.Text"), "BoolText.TextColor"=u32 0 ("Boolean Text.Colors:FG Color")) -> ()  [unwired: 2 in, 2 out]
                n175 = call "HT3_Finish.vi"("FileHeaderPos"=w476, "Rates"=w473, "Stop Reason"=w478, "error in"=w482, "Num Records"=w479, "Stop After (ms)"=w468, "refnum in"=w480) -> ("error out"=w481:errorcluster)  [unwired: 4 in]
                n176 = Merge Errors(w467, w466) -> (w465:errorcluster)
              }
            }
            n177 = local read "Laser  Profile"() -> (w369:string)
            n178 = String To Byte Array(string=w369) -> (unsigned byte array=w367:u8[])
            n179 = Subtract(x=w367, y=48) -> (x-y=w362:i32[])
            n180 = String Length(string=w369) -> (length=w359:i32)
            n181 = Initialize Array(0, 5, 2) -> (w363:i32[][])
            n182 = Replace Array Subset(array=w363, new element=w362, index (col)=w355) -> (w361:i32[][])  [unwired: 1 in]
            n183 = Array Subset(array=w360, index=w355, length=w359) -> (w358:i32[])
            n184 = Replace Array Subset(array=w361, new element=w358, index (col)=1) -> (w357:i32[][])  [unwired: 1 in]
            n185 = call "HT3_Create.vi"("Laser"=w357, "Save pt3"=w349, "error in"=w397, "Comment"=w412, "ht3 Header in"=w399, "File Path"=w403) -> ("error out"=w338:errorcluster, "FileHeaderPos"=w382:T23, "refnum out"=w408:refnum<file>)  [unwired: 3 in]
            n186 = call "HH_Start.vi"("Device Index"=w340, "Acq. Time"=w294, "error in (no error)"=w338) -> ("error out"=w308:errorcluster)  [unwired: 11 in, 1 out]
            n187 = case shown="True" w309 {
              tunnel: [w434 w438] -> w288
              tunnel: w338 -> [w434 w437]
              tunnel: w292 -> [_ w436]
              tunnel: [_ w435] -> w297
              frame False {
              }
              frame True {
                n188 = control-ref of="NxtAutMesPoint"() -> (w443:refnum<vi>)
                n189 = control-ref of="Workspace"() -> (w444:refnum<vi>)
                n190 = control-ref of="y-position"() -> (w440:refnum<vi>)
                n191 = control-ref of="x-position"() -> (w441:refnum<vi>)
                n192 = control-ref of="z-position"() -> (w439:refnum<vi>)
                n193 = control-ref of="Pattern"() -> (w442:refnum<vi>)
                n194 = call "DefocussedImage.vi"("Path in"=w444, "reference"=w443, "Boolean"=w436, "reference 2"=w442, "reference 3"=w441, "error in (no error)"=w437, "reference 4"=w440, "reference 5"=w439) -> ("camout"=w435:i32[], "error out"=w438:errorcluster)  [unwired: 6 in]
              }
            }
            n195 = Unbundle By Name(w308) -> ("status"=w420:bool)
            n196 = Not(x=w420) -> (.not. x?=w419:bool)
            n197 = case shown="True" w419 {
              tunnel: [w509 w512] -> w307
              tunnel: w308 -> [w510 w521]
              tunnel: w305 -> [w511 w532]
              tunnel: [w511 w531] -> w418
              tunnel: w340 -> [w504 w520]
              tunnel: w415 -> [_ w528]
              tunnel: w383 -> [_ w527]
              tunnel: [w508 w526] -> w414
              tunnel: [w508 w525] -> w413
              tunnel: w408 -> [w507 w524]
              tunnel: [w507 w523] -> w407
              tunnel: [i64 0 ("Num Records Total") w522] -> w406
              tunnel: [dbl[] [] w517] -> w375
              tunnel: [0 w516] -> w374
              frame False {
                w508 = FALSE ("Stop Measurement")
                n198 = call "HH_Stop.vi"("Device Index"=w504, "error in (no error)"=w510) -> ("error out"=w509:errorcluster)  [unwired: 12 in, 1 out]
              }
              frame True {
                # "Overflow Interv. Time (s)"
                # "No Error"
                n199 = Initialize Array(0, 5) -> (w515:i32[])
                n200 = while {
                  tunnel: w520 -> [w541]
                  tunnel: w528 -> [w565]
                  tunnel: w527 -> [w564]
                  shift-right: [w542] -> w530
                  shift-left: w521 -> [w566]
                  shift-right: [w563] -> w531
                  shift-left: w532 -> [w563]
                  shift-right: [FALSE ("Reset")] -> _
                  shift-left: TRUE ("Reset") -> [w559]
                  tunnel: [w556] -> w526
                  tunnel: [w548] -> w525
                  tunnel: w524 -> [w552]
                  tunnel: [w551] -> w523
                  tunnel: [w550] -> w522
                  tunnel: [w549] -> w516
                  shift-right: [w536] -> w518
                  shift-left: w515 -> [w535]
                  tunnel: [w533] -> w519
                  i -> [w534]
                  stop <- w562 stop-if-true
                  n201 = call "HH_FIFORead.vi"("Device Index"=w541, "Buffer In"=w565, "Count"=w564, "error in (no error)"=w566) -> ("OK"=w557:bool, "Buffer Out"=w553:u32[], "Data Count"=w554:i32, "FiFo Overrun"=w556:bool, "error out"=w555:errorcluster)  [unwired: 7 in]
                  n202 = Wait (ms)(milliseconds to wait=u32 10) -> ()  [unwired: 1 out]
                  n203 = local write "Buffer Overrun"(w556) -> ()
                  n204 = Unbundle(w555) -> ("status"=w561:bool)  [unwired: 2 out]
                  n205 = call "HT3_Write.vi"("error in"=w555, "Data Count"=w554, "Data in"=w553, "refnum in"=w552) -> ("error out"=w543:errorcluster, "refnum out"=w551:refnum<file>)  [unwired: 6 in]
                  n206 = call "HH_TraceAndHisto.vi"("Data In"=w553, "Reset"=w559, "Data Count"=w554) -> ("Histograms"=w545:i32[][], "Total Oveflow Count"=w549:u64, "Num Records Total"=w550:i64, "Traces"=w544:i32[][])  [unwired: 8 in, 1 out]
                  n207 = local read "Stop Measurement"() -> (w547:bool)
                  n208 = local read "Global Stop"() -> (w546:bool)
                  n209 = local write "Trace"(w544) -> ()
                  n210 = call "GetCountRates.vi"("error in (no error)"=w543, "DeviceIndex"=w541) -> ("error out"=w542:errorcluster, "CntRates"=w537:dbl[], "SyncRate"=w538:i32)  [unwired: 1 in]
                  n211 = local write "Histogram"(w545) -> ()
                  n212 = Compound Arithmetic op=OR(invert w557, w561, w546, w547) -> (w562:bool)
                  n213 = Insert Into Array(array=w537, index=0, new element=w538) -> (w539:dbl[])
                  n214 = Or(x=w547, y=w546) -> (x .or. y?=w548:bool)
                  n215 = Add(x=w535, y=w539) -> (x+y=w536:dbl[])
                  n216 = Increment(x=w534) -> (x+1=w533:i32)
                }
                n217 = Divide(x=w518, y=w519) -> (x/y=w517:dbl[])
                n218 = call "HH_Stop.vi"("Device Index"=w520, "error in (no error)"=w530) -> ("error out"=w512:errorcluster)  [unwired: 12 in, 1 out]
              }
            }
            n219 = Reshape Array(w297, w296, w295) -> (w289:i32[][])
            n220 = property on="Point" class="IntGraph (strict)"(error in=w288, "Value"=w289) -> (error out=w287:errorcluster)  [unwired: 1 in, 1 out]
            n221 = Merge Errors(w307, w287) -> (w306:errorcluster)
            n222 = call "AOTF-Trigger_1.vi"("Channel"=w369, "Pulse length"=w360, "Sync trigger ratio"=5, "error in (no error)"=w304, "Triggered"=FALSE) -> ("error out"=w378:errorcluster)  [unwired: 2 in]
            n223 = call "MOV.vi"("System no."=w335, "Axes to move"=w329, "Position values"=w328, "error in"=w353) -> ("error out"=w352:errorcluster)  [unwired: 15 in]
          }
          frame "Save Color Image" {
            n224 = local read "Active pt3"() -> (w574:path)
            n225 = call "MTS_GetFileFromWS.vi"(".pt3 File Name"=w574) -> ("File Header"=w573:T25)  [unwired: 9 in, 1 out]
            n226 = Unbundle By Name(w573) -> ("Measurement Type"=w572:T26, "Pixels"=w569:i32[])
            n227 = control-ref of="WS File Tree"() -> (w575:refnum<vi>)
            n228 = Equal?(x=T13."Image File" ("Measurement Type"), y=w572) -> (x = y?=w570:bool)
            n229 = case shown="True" w570 {
              tunnel: w578 -> [w579 w602]
              tunnel: w574 -> [_ w601]
              tunnel: w574 -> [_ _]
              tunnel: [w579 w581] -> w567
              tunnel: w575 -> [_ _]
              tunnel: w569 -> [_ w586]
              frame False {
              }
              frame True {
                # "Image Intensity Array"
                # "Image Intensity Array"
                n230 = call "HT3_Open.vi"("error in"=w602, "File Path"=w601) -> ("error out"=w594:errorcluster, "Header"=w598:T27, "refnum out"=w600:refnum<file>)  [unwired: 3 in, 4 out]
                n231 = Unbundle By Name(w598) -> ()  [unwired: 15 out]
                n232 = Index Array(array=w586, index #2=1 ("index")) -> (element #1=w583:i32, element #2=w584:i32)  [unwired: 1 in]
                n233 = Initialize Array(0 ("element"), w583, w584) -> (w596:i32[][])
                n234 = Initialize Array(0 ("element"), 4 ("dimension size"), w583, w584) -> (w589:i32[][][])
                n235 = while {
                  tunnel: w600 -> [w627]
                  shift-right: [FALSE ("Start From Top")] -> _
                  shift-left: TRUE ("Start From Top") -> [w621]
                  shift-right: [w620] -> w593
                  shift-left: w594 -> [w618]
                  tunnel: [w619] -> w592
                  tunnel: w596 -> [w617]
                  tunnel: [w616] -> w595
                  tunnel: [w617] -> _
                  stop <- w624 stop-if-true
                  n236 = call "HT3_Read.vi"("Start From Top"=w621, "error in"=w618, "Data count"=10000, "refnum in"=w627) -> ("error out"=w620:errorcluster, "Data out"=w623:u32[], "refnum out"=w619:refnum<file>, "EOF?"=w624:bool)  [unwired: 4 in]
                  n237 = Array Size(array=w623) -> (size(s)=w622:i32)
                  n238 = call "HH_FileToImage_1.vi"("Data In"=w623, "Reset"=w621, "Data Count"=w622) -> ("Histograms"=w616:i32[][])  [unwired: 7 in, 5 out]
                }
                n239 = call "MTS_SelectTCSPCBinning.vi"("Histograms in"=w595) -> ("TCSPC Binning"=w588:i32[][])  [unwired: 1 in, 9 out]
                n240 = while {
                  tunnel: w592 -> [w615]
                  shift-right: [FALSE ("Start From Top")] -> _
                  shift-left: TRUE ("Start From Top") -> [w609]
                  shift-right: [w608] -> w580
                  shift-left: w593 -> [w604]
                  tunnel: [w607] -> w582
                  tunnel: w589 -> [w606]
                  tunnel: [w605] -> _
                  tunnel: w588 -> [w603]
                  stop <- w612 stop-if-true
                  n241 = call "HT3_Read.vi"("Start From Top"=w609, "error in"=w604, "Data count"=10000, "refnum in"=w615) -> ("error out"=w608:errorcluster, "Data out"=w611:u32[], "refnum out"=w607:refnum<file>, "EOF?"=w612:bool)  [unwired: 4 out]
                  n242 = Array Size(array=w611) -> (size(s)=w610:i32)
                  n243 = call "HH_ToColorImage.vi"("Data In"=w611, "Reset"=w609, "Image Array In"=w606, "Data Count"=w610, "TCSPC Binning"=w603) -> ("Image Array Out"=w605:i32[][][])  [unwired: 2 in, 8 out]
                }
                n244 = Close File(refnum=w582, error in=w580) -> (error out=w581:errorcluster)  [unwired: 1 out]
              }
            }
          }
          frame "Find Single Mol." {
            # "dirty trick"
            n245 = local read "Active pt3"() -> (w654:path)
            n246 = call "MTS_GetFileFromWS.vi"(".pt3 File Name"=w654) -> ("File Header"=w653:T25)  [unwired: 9 in, 1 out]
            n247 = Unbundle By Name(w653) -> ("Measurement Type"=w652:T26, "Pixels"=w640:i32[], "Upper Left"=w649:T28, "Scan Axis"=w648:enum32{"x-y", "x-z", "y-z"})
            n248 = local read "Picture size 2"() -> (w635:dbl)
            n249 = local read "Picture size"() -> (w638:dbl)
            n250 = local read "Resolution"() -> (w636:dbl)
            n251 = local read "X-Position"() -> (w629:dbl)
            n252 = local read "Y-Position"() -> (w628:dbl)
            n253 = Divide(x=w638, y=w636) -> (x/y=w637:dbl)
            n254 = Divide(x=w635, y=w636) -> (x/y=w634:dbl)
            n255 = Equal?(x=T13."Image File" ("Measurement Type"), y=w652) -> (x = y?=w650:bool)
            n256 = call "MTS_ScannerXYZToImageXY.vi"("Axis"=w648, "Scanner XYZ"=w649) -> ("Image Y"=w631:dbl, "Image X"=w633:dbl)
            n257 = case shown="True" TRUE {
              tunnel: [w657 w660] -> w639
              tunnel: w640 -> [w657 _]
              tunnel: w637 -> [_ w664]
              tunnel: w634 -> [_ w663]
              tunnel: [w656 w659] -> w632
              tunnel: w633 -> [w656 _]
              tunnel: [w655 w658] -> w630
              tunnel: w631 -> [w655 _]
              tunnel: w629 -> [_ w659]
              tunnel: w628 -> [_ w658]
              frame False {
              }
              frame True {
                n258 = To Long Integer(number=w664) -> (32bit integer=w662:i32)
                n259 = To Long Integer(number=w663) -> (32bit integer=w661:i32)
                n260 = Build Array(w662, w661) -> (w660:i32[])
              }
            }
            n261 = Build Array(w638, w635) -> (w644:dbl[])
            n262 = case shown="True" w650 {
              tunnel: w647 -> [w665 w740]
              tunnel: w654 -> [_ _]
              tunnel: w654 -> [_ _]
              tunnel: [w665 w745] -> w645
              tunnel: w639 -> [_ w762]
              tunnel: w644 -> [_ w744]
              tunnel: w632 -> [_ w754]
              tunnel: w630 -> [_ w755]
              frame False {
              }
              frame True {
                w714 = T4 1 items=["Center of Mass X", "Center of Mass Y", "First Pixel X", "First Pixel Y", "Bounding Rect Left", "Bounding Rect Top", "Bounding Rect Right", "Bounding Rect Bottom", "Max Feret Diameter Start X", "Max Feret Diameter Start Y", "Max Feret Diameter End X", "Max Feret Diameter End Y", "Max Horiz. Segment Length Left", "Max Horiz. Segment Length Right", "Max Horiz. Segment Length Row", "-", "Bounding Rect Width", "Bounding Rect Height", "Bounding Rect Diagonal", "Perimeter", "Convex Hull Perimeter", "Holes' Perimeter", "Max Feret Diameter", "Equivalent Ellipse Major Axis", "Equivalent Ellipse Minor Axis", "Equivalent Ellipse Minor Axis (Feret)", "Equivalent Rect Long Side", "Equivalent Rect Short Side", "Equivalent Rect Diagonal", "Equivalent Rect Short Side (Feret)", "Average Horiz. Segment Length", "Average Vert. Segment Length", "Hydraulic Radius", "Waddel Disk Diameter", "-", "Area", "Holes' Area", "Particle & Holes' Area", "Convex Hull Area", "Image Area", "-", "Number of Holes", "Number of Horiz. Segments", "Number of Vert. Segments", "-", "Orientation", "Max Feret Diameter Orientation", "-", "% Area/Image Area", "% Area/(Particle & Holes' Area)", "Ratio of Equivalent Ellipse Axes", "Ratio of Equivalent Rect Sides", "-", "Elongation Factor", "Compactness Factor", "Heywood Circularity Factor", "Type Factor", "-", "Sum X", "Sum Y", "Sum XX", "Sum XY", "Sum YY", "Sum XXX", "Sum XXY", "Sum XYY", "Sum YYY", "-", "Moment of Inertia XX", "Moment of Inertia XY", "Moment of Inertia YY", "Moment of Inertia XXX", "Moment of Inertia XXY", "Moment of Inertia XYY", "Moment of Inertia YYY", "Norm. Moment of Inertia XX", "Norm. Moment of Inertia XY", "Norm. Moment of Inertia YY", "Norm. Moment of Inertia XXX", "Norm. Moment of Inertia XXY", "Norm. Moment of Inertia XYY", "Norm. Moment of Inertia YYY", "Hu Moment 1", "Hu Moment 2", "Hu Moment 3", "Hu Moment 4", "Hu Moment 5", "Hu Moment 6", "Hu Moment 7"] ("Measurement Parameter")
                w695 = TRUE ("Measurement Type")
                w719 = T4 0 items=["Center of Mass X", "Center of Mass Y", "First Pixel X", "First Pixel Y", "Bounding Rect Left", "Bounding Rect Top", "Bounding Rect Right", "Bounding Rect Bottom", "Max Feret Diameter Start X", "Max Feret Diameter Start Y", "Max Feret Diameter End X", "Max Feret Diameter End Y", "Max Horiz. Segment Length Left", "Max Horiz. Segment Length Right", "Max Horiz. Segment Length Row", "-", "Bounding Rect Width", "Bounding Rect Height", "Bounding Rect Diagonal", "Perimeter", "Convex Hull Perimeter", "Holes' Perimeter", "Max Feret Diameter", "Equivalent Ellipse Major Axis", "Equivalent Ellipse Minor Axis", "Equivalent Ellipse Minor Axis (Feret)", "Equivalent Rect Long Side", "Equivalent Rect Short Side", "Equivalent Rect Diagonal", "Equivalent Rect Short Side (Feret)", "Average Horiz. Segment Length", "Average Vert. Segment Length", "Hydraulic Radius", "Waddel Disk Diameter", "-", "Area", "Holes' Area", "Particle & Holes' Area", "Convex Hull Area", "Image Area", "-", "Number of Holes", "Number of Horiz. Segments", "Number of Vert. Segments", "-", "Orientation", "Max Feret Diameter Orientation", "-", "% Area/Image Area", "% Area/(Particle & Holes' Area)", "Ratio of Equivalent Ellipse Axes", "Ratio of Equivalent Rect Sides", "-", "Elongation Factor", "Compactness Factor", "Heywood Circularity Factor", "Type Factor", "-", "Sum X", "Sum Y", "Sum XX", "Sum XY", "Sum YY", "Sum XXX", "Sum XXY", "Sum XYY", "Sum YYY", "-", "Moment of Inertia XX", "Moment of Inertia XY", "Moment of Inertia YY", "Moment of Inertia XXX", "Moment of Inertia XXY", "Moment of Inertia XYY", "Moment of Inertia YYY", "Norm. Moment of Inertia XX", "Norm. Moment of Inertia XY", "Norm. Moment of Inertia YY", "Norm. Moment of Inertia XXX", "Norm. Moment of Inertia XXY", "Norm. Moment of Inertia XYY", "Norm. Moment of Inertia YYY", "Hu Moment 1", "Hu Moment 2", "Hu Moment 3", "Hu Moment 4", "Hu Moment 5", "Hu Moment 6", "Hu Moment 7"] ("Measurement Parameter")
                w734 = T29 4 items=["Grayscale (U8)", "Grayscale (I16)", "Grayscale (SGL)", "Complex (CSG)", "RGB (U32)", "HSL (U32)", "RGB (U64)", "Grayscale (U16)"] ("Image Type")
                w742 = T29 4 items=["Grayscale (U8)", "Grayscale (I16)", "Grayscale (SGL)", "Complex (CSG)", "RGB (U32)", "HSL (U32)", "RGB (U64)", "Grayscale (U16)"] ("Image Type")
                w761 = 1 ("index")
                # "Pixel Size [um]"
                n263 = Index Array(array=w744, index #2=w761) -> (element #1=w760:dbl, element #2=w757:dbl)  [unwired: 1 in]
                n264 = Index Array(array=w762, index #2=w761) -> (element #1=w759:i32, element #2=w758:i32)  [unwired: 1 in]
                n265 = Divide(x=w760, y=w759) -> (x/y=w670:dbl)
                n266 = Divide(x=w757, y=w758) -> (x/y=w756:dbl)
                n267 = Reciprocal(x=w670) -> (1/x=w671:dbl)
                n268 = Multiply(x=w671, y="Focuswidth") -> (x*y=w669:dbl)
                n269 = Random Number (0-1)() -> (number: 0 to 1=w739:dbl)
                n270 = Number To Decimal String(number=w739) -> (decimal integer string=w738:string)  [unwired: 1 in]
                n271 = Concatenate Strings(w738, "IMAQ CreatePatternimg" ("Image Name")) -> (w736:string)
                n272 = call "IMAQ Create"("Image Name"=w736, "Image Type"=w742, "error in (no error)"=w740) -> ("New Image"=w741:T2, "error out"=w729:errorcluster)  [unwired: 2 in]
                n273 = local read "Image"() -> (w673:i32[][])
                n274 = call "MTS_IntensityArrayToImage.vi"(0:"Image"=w741, 1:"Image"=w673, "error in (no error)"=w729, "Log Scale"=FALSE) -> ("Image Out"=w694:T2, "error out"=w686:errorcluster)  [unwired: 10 in]
                n275 = Random Number (0-1)() -> (number: 0 to 1=w733:dbl)
                n276 = Array To Cluster(array=T19 [] ("MesaurementSelection")) -> (cluster=w722:T30)
                n277 = Number To Decimal String(number=w733) -> (decimal integer string=w732:string)  [unwired: 1 in]
                n278 = Unbundle By Name(w722) -> ("MesaurementSelection[0]"=w720:T31, "MesaurementSelection[1]"=w715:T31, "MesaurementSelection[2]"=w710:T31, "MesaurementSelection[3]"=w701:T31)
                n279 = Concatenate Strings(w732, "IMAQ CreatePatternimg2" ("Image Name")) -> (w730:string)
                n280 = call "IMAQ Create"("Image Name"=w730, "Image Type"=w734, "error in (no error)"=w686) -> ("New Image"=w728:T2, "error out"=w685:errorcluster)  [unwired: 2 in]
                n281 = Bundle By Name(cluster=w720, "Measurement Parameter"=w719, "Range Lower Value"="X Start 2", "Range Upper Value"="X End 2", "Range"="Exclude / Include X", "Measurement Type"=w695) -> (w709:T31)
                n282 = Bundle By Name(cluster=w715, "Measurement Parameter"=w714, "Range Lower Value"="Y Start 2", "Range Upper Value"="Y End 2", "Range"="Exclude / Include Y", "Measurement Type"=w695) -> (w708:T31)
                n283 = Bundle By Name(cluster=w710, "Measurement Parameter"="Measurement Parameter 1", "Range Lower Value"="Range Lower Value Par 1", "Range Upper Value"="Range Upper Value  Par 1", "Range"="Ex/In Par 1", "Measurement Type"=w695) -> (w707:T31)
                n284 = Bundle By Name(cluster=w701, "Measurement Parameter"="Measurement Parameter 2", "Range Lower Value"="Range Lower Value Par 2", "Range Upper Value"="Range Upper Value Par 2", "Range"="Ex/In Par 2", "Measurement Type"=w695) -> (w700:T31)
                n285 = Build Array(w709, w708, w707, w700) -> (w706:T19)
                n286 = call "MTS_IntensityArrayToImage.vi"(0:"Image"=w728, 1:"Image"=w673, "error in (no error)"=w685, "Log Scale"=TRUE) -> ("Image Out"=w679:T2, "error out"=w684:errorcluster)  [unwired: 10 in]
                n287 = case shown="0, Default" "Detection Modus" {
                  tunnel: "Remove Outliers" -> [_ w794]
                  tunnel: [w771 w785] -> w735
                  tunnel: w684 -> [w776 w793]
                  tunnel: [w769 w783] -> w726
                  tunnel: "Filter" -> [_ w792]
                  tunnel: w706 -> [_ w791]
                  tunnel: w694 -> [_ w786]
                  tunnel: path "C:/Users/Core-FCS/Desktop/Documents/AbelFCS/ParticleFinder/SingleMoleculePatternFinder/Patterns/azimutalGolden.png" ("Template File Path (GeometricMatching)") -> [_ _]
                  tunnel: "Settings (GeometricMatching)" -> [_ _]
                  tunnel: IMAQ_Rounding_Mode."Optimize" ("Rounding Mode Gaussian") -> [_ w790]
                  tunnel: IMAQ_Rounding_Mode."Optimize" ("Rounding Mode Convolution") -> [_ w789]
                  tunnel: "Square/Hexa" -> [_ w788]
                  tunnel: "Connectivity 4/8" -> [_ w787]
                  tunnel: w679 -> [w773 w781]
                  tunnel: [w773 w778] -> w683
                  tunnel: [w775 w779] -> w681
                  tunnel: "Manual" -> [_ w777]
                  tunnel: w673 -> [w767 _]
                  tunnel: "Mode" -> [w766 _]
                  tunnel: w669 -> [w765 _]
                  tunnel: [w764 _] -> w667
                  tunnel: "NA" -> [w763 _]
                  frame 0, Default {
                    n288 = To Double Precision Float(number=w767) -> (double precision float=w768:dbl[][])
                    n289 = script code="addpath(path);\nswitch (mode)\ncase 0\nmaskGauss = GenGauss2D(focus);\n[err,bim,cim,sim,yc,xc,bc,cc,sc,len,imm]=FindPatternCP(image,maskGauss,[],[],[],1.5);\npattern=maskGauss;\ncase 1\nmaskRad=Radialpattern_gen('radial', focus,NA);\n[err,bim,cim,sim,yc,xc,bc,cc,sc,len,imm]=FindPatternCP(image,maskRad,[],[],[],1);\npattern=maskRad(:,:,15);\ncase 2\nmaskAzi=Radialpattern_gen('azimuthal', focus,NA);\n[err,bim,cim,sim,yc,xc,bc,cc,sc,len,imm]=FindPatternCP(image,maskAzi,[],[],[],1.5);\npattern=maskAzi(:,:,15);\nend\nxc=xc-1;\nyc=yc-1;"("??"=w776, "path"="C:\\Users\\Core-FCS\\Desktop\\Documents\\CoreSetupNew\\MatlabLibAbelFCS", "image"=w768, "mode"=w766, "focus"=w765, "NA"=w763) -> ("??"=w775:errorcluster, "pattern"=w764:dbl[][], "xc"=w772:dbl[], "yc"=w770:dbl[])
                    n290 = Build Array(w772, w770) -> (w771:dbl[][])
                    n291 = Array Size(array=w770) -> (size(s)=w769:i32)
                  }
                  frame 1 {
                    n292 = call "SingleMoleFinderEasy.vi"("Image Src"=w786, "Number of Erosion"=w794, "HolesBorder"=w792, "Selection Values"=w791, "Rounding Mode Gaussian"=w790, "error in"=w793, "Rounding Mode Convolution"=w789, "Square/Hexa (Square)"=w788, "Connectivity 4/8 (8)"=w787) -> ("Number of Particles"=w782:i32, "Particle Measurements (Pixels)"=w784:dbl[][], "error out"=w780:errorcluster)  [unwired: 15 in, 1 out]
                    n293 = case shown="True" w777 {
                      tunnel: w780 -> [w798 w806]
                      tunnel: [w798 w805] -> w779
                      tunnel: [w795 w804] -> w778
                      tunnel: [w796 w803] -> w785
                      tunnel: w784 -> [w796 w800]
                      tunnel: [w797 w802] -> w783
                      tunnel: w782 -> [w797 w801]
                      tunnel: w781 -> [w795 w799]
                      frame False {
                      }
                      frame True {
                        n294 = while {
                          tunnel: w806 -> [w821]
                          tunnel: [w820] -> w805
                          tunnel: w799 -> [w819]
                          tunnel: [w818] -> w804
                          shift-right: [w811] -> w803
                          shift-left: w800 -> [w810]
                          tunnel: [w809] -> w802
                          tunnel: w801 -> [w808]
                          i -> [w815]
                          stop <- w817 stop-if-true
                          n295 = call "IMAQ Select Point"("Window Number (0...15)"=1, "error in (no error)"=w821, "Image In"=w819) -> ("error out"=w820:errorcluster, "Cancelled"=w817:bool, "Point"=w816:T32, "Image Out (duplicate)"=w818:T2)  [unwired: 5 in]
                          n296 = Unbundle(w816) -> ("X"=w814:sgl, "Y"=w813:sgl)
                          n297 = Build Array(w814, w813) -> (w812:sgl[])
                          n298 = Add(x=w808, y=w815) -> (x+y=w809:i32)
                          n299 = Insert Into Array(array=w810, index (row)=w809, new element=w812) -> (w811:dbl[][])  [unwired: 1 in]
                        }
                      }
                    }
                  }
                }
                "Number of Particles" <- w726
                "Image 2" <- w667
                n300 = Index Array(array=w735, index (col) #1=0 ("index (row)"), index (col) #2=1 ("index (col)")) -> (element #1=w678:dbl[], element #2=w676:dbl[])  [unwired: 2 in]
                n301 = Multiply(x=w670, y=w678) -> (x*y=w753:dbl[])
                n302 = Multiply(x=w676, y=w756) -> (x*y=w752:dbl[])
                n303 = To Word Integer(number=w678) -> (16bit integer=w677:i16[])
                n304 = To Word Integer(number=w676) -> (16bit integer=w675:i16[])
                n305 = Add(x=w754, y=w753) -> (x+y=w748:dbl[])
                n306 = Add(x=w752, y=w755) -> (x+y=w747:dbl[])
                n307 = for {
                  N: w726 -> [_]
                  shift-right: [w828] -> w682
                  shift-left: w683 -> [w829]
                  tunnel: w677 -> [w827] mode=indexing
                  tunnel: w675 -> [w826] mode=indexing
                  shift-right: [w830] -> w680
                  shift-left: w681 -> [w831]
                  tunnel: u32 16738560 -> [w825]
                  tunnel: 3.0 ("x") -> [w824]
                  n308 = call "MTS_DrawCrossIMAQIamge.vi"("Image"=w829, "Size"=w824, "Color"=w825, "X"=w827, "Y"=w826, "error in (no error)"=w831) -> ("Image Out"=w828:T2, "error out"=w830:errorcluster)  [unwired: 8 in]
                }
                "AM image" <- w682
                n309 = Build Array(w748, w747, w677, w675) -> (→"Pattern":dbl[][])
                n310 = global write "patternImg.vi" "New Image"(w682) -> ()
                n311 = flat-sequence {
                  tunnel: w680 -> [w823]
                  tunnel: [w823] -> w745
                  frame #0 {
                    n312 = local write "Tab Control"(T1."AutoMesaurement" ("Tab Control")) -> ()
                  }
                }
              }
            }
          }
          frame "Auto Measurement Control" {
            # "Init"
            n313 = local read "Pattern"() -> (w842:dbl[][])
            n314 = Index Array(array=w842, index (row) #1=2 ("index (row)"), index (row) #2=3 ("index (col)")) -> (element #1=w839:dbl[], element #2=→"subarray":dbl[])  [unwired: 2 in]
            n315 = local read "NxtAutMesPoint"() -> (w850:i32)
            n316 = Array Size(array=w839) -> (size(s)=w838:i32)
            n317 = Less Than 0?(x=w850) -> (x < 0?=w853:bool)
            n318 = case shown="False" w853 {
              tunnel: w847 -> [w874 w878]
              tunnel: [w874 w877] -> w851
              tunnel: [w873 w875] -> w849
              tunnel: w838 -> [_ w875]
              frame False {
                n319 = local read "Auto Measure Points"() -> (w873:i32)
              }
              frame True {
                n320 = Number To Decimal String(number=w875) -> (decimal integer string=w880:string)  [unwired: 1 in]
                n321 = Concatenate Strings("Point 1 / " ("Caption.Text"), w880) -> (w879:string)
                n322 = property on="Auto Meas Progress" class="Slide (strict)"(error in=w878, "Scale.Minimum"=0.0 ("Scale.Range:Minimum"), "Scale.Maximum"=w875, "Value"=1 ("Auto Meas Progress"), "Caption.Text"=w879) -> (error out=w877:errorcluster)  [unwired: 1 in, 1 out]
                "Auto Measure Points" <- w875
              }
            }
            n323 = Increment(x=w850) -> (x+1=w833:i32)
            "NxtAutMesPoint" <- w833
            n324 = Greater Or Equal?(x=w833, y=w849) -> (x >= y?=w852:bool)
            n325 = Increment(x=w833) -> (x+1=w848:i32)
            n326 = Index Array(array=w842, index (row) #1=2 ("index (row)"), index (col) #1=w833, index (row) #2=3 ("index (col)"), index (col) #2=w833) -> (element #1=w841:dbl, element #2=w840:dbl)
            n327 = case shown="False" w852 {
              tunnel: w851 -> [w864 w872]
              tunnel: [w870 w872] -> w845
              tunnel: [T17."Auto Point" ("Do Measurement") T17."No Measurement" ("Do Measurement")] -> w844
              tunnel: w848 -> [w865 _]
              tunnel: w841 -> [w862 _]
              tunnel: w840 -> [w861 _]
              tunnel: w849 -> [w858 _]
              frame False {
                # "Prpare For Next Point"
                # "1 loc max  2 undef 0 saddle -1 local min"
                n328 = global read "patternImg.vi" "New Image"() -> (w854:T2)
                n329 = Number To Decimal String(number=w865) -> (decimal integer string=w867:string)  [unwired: 1 in]
                n330 = Number To Decimal String(number=w858) -> (decimal integer string=w859:string)  [unwired: 1 in]
                n331 = Concatenate Strings("Point " ("Caption.Text"), w867, " / " ("Caption.Text"), w859) -> (w866:string)
                n332 = call "MTS_DrawCrossIMAQIamge.vi"("Image"=w854, "Size"=3.0 ("x"), "Color"=u32 6618880, "X"=w862, "Y"=w861, "error in (no error)"=w864) -> ("Image Out"=w855:T2, "error out"=w863:errorcluster)  [unwired: 8 in]
                n333 = local write "AM image"(w855) -> ()
                n334 = property on="Auto Meas Progress" class="Slide (strict)"(error in=w863, "Value"=w865, "Caption.Text"=w866) -> (error out=w870:errorcluster)  [unwired: 1 in, 1 out]
              }
              frame True {
                # "No More Points"
              }
            }
          }
        }
        n335 = local write "Buffer Overrun"(w22) -> ()
      }
      frame Error {
      }
    }
    n336 = Unbundle(w7) -> ("status"=w6:bool)  [unwired: 2 out]
    n337 = flat-sequence {
      tunnel: w10 -> [w898]
      tunnel: [w898] -> w9
      tunnel: w5 -> [w895]
      frame #0 {
        n338 = local write "Task"(w895) -> ()
        n339 = Equal?(x=w895, y=T9."No Measurement" ("Do Measurement")) -> (x = y?=w896:bool)
        n340 = Not(x=w896) -> (.not. x?=w897:bool)
        n341 = local write "Running"(w897) -> ()
      }
    }
    n342 = local read "Global Stop"() -> (w13:bool)
    n343 = Compound Arithmetic op=OR(w6, w11, w13) -> (w12:bool)
  }
